vi "MoD Main-Optimize - HPLC PhotoRedox.vi"() -> ()   [LabVIEW 2015]
uses:
  <vilib>/silver_ctls/ArrayMatrixCluster/Real Matrix NI_Silver.ctl
  <vilib>/ni845x/ni845x.llb/ni845xControl.ctl
  <vilib>/MakerHub/LINX/Public/Peripherals/Analog/Analog Read 1 Chan.vi
  <vilib>/MakerHub/LINX/Public/Peripherals/Analog/Analog Read N Chans.vi
  <vilib>/MakerHub/LINX/Public/Peripherals/PWM/PWM Set Duty Cycle 1 Chan.vi
  <vilib>/MakerHub/LINX/Public/Peripherals/Digital/Digital Write 1 Chan.vi
  <vilib>/MakerHub/LINX/Private/Local IO/LinxAnalogRead.vi
  <vilib>/MakerHub/LINX/Public/Utilities/Check Channel.vi
  <vilib>/MakerHub/LINX/Public/Peripherals/Digital/Digital Write N Chans.vi
  <vilib>/MakerHub/LINX/Private/Local IO/LinxDigitalWrite.vi
  <vilib>/addons/control/pid/pid.llb/PID Control Input Filter (DBL).vi
  <vilib>/MakerHub/LINX/Private/Utilties/Generate Error.vi
  <vilib>/addons/control/pid/autopid.llb/PID Online Autotuning (Relay Feedback).vi
  <vilib>/Analysis/Matrix/Numeric/Conversions/Array To Matrix - RA2.vi
  <vilib>/MakerHub/LINX/Public/Peripherals/PWM/PWM Set Duty Cycle N Chans.vi
  <vilib>/ni845x/ni845x.llb/NI-845x Close Device Reference.vi
  <vilib>/addons/control/pid/NI_PID_autopid.lvlib
  <vilib>/addons/control/pid/NI_PID_pid.lvlib
  <vilib>/Analysis/Matrix/NI_Matrix.lvlib
  <vilib>/MakerHub/LINX/LMH-LINX.lvlib
  <instrlib>/Harvard Apparatus PHD Ultra Series/Harvard Apparatus PHD Ultra Series.lvlib
panel:
  out "running?":bool=TRUE
  out "new_reactor_volume":bool[](array[boolean])
  out "new_reactor_length":bool[](array[boolean])
  out "Phase_Sensor_voltage":dbl
  out "P_tot":dbl
  out "pause for ms":bool=TRUE
  out "stop_xl_write":bool=TRUE
  out "Num_exp_till_pause":i32
  out "Syringe_pump?":bool=TRUE
  out "System Error":bool=TRUE
  out "error out":errorcluster
  out "Pump setpoint(ul/min) 6":dbl format="%#_13g"
  out "Pump setpoint(ul/min) 5":dbl format="%#_13g"
  out "Pump setpoint(ul/min) 4":dbl format="%#_13g"
  out "Pump setpoint(ul/min) 3":dbl format="%#_13g"
  out "Pump setpoint(ul/min) 2":dbl format="%#_13g"
  out "Pump setpoint(ul/min) 1":dbl format="%#_13g"
  out "Volume (ul) 5":dbl format="%#_13g"
  out "Volume (ul) 4":dbl format="%#_13g"
  out "Volume (ul) 3":dbl format="%#_13g"
  out "Volume (ul) 2":dbl format="%#_13g"
  out "Volume (ul) 1":dbl format="%#_13g"
  in  "tau 5":dbl format="%#_13g"
  out "tau 4":dbl format="%#_13g"
  out "tau 3":dbl format="%#_13g"
  out "tau 2":dbl format="%#_13g"
  out "tau 1":dbl format="%#_13g"
  out "Reactor Length":dbl format="%#_13g"
  out "Flowrate Sensor 2":dbl format="%#_13g"
  out "Flowrate Sensor 1":dbl format="%#_13g"
  out "Pressure 2":dbl format="%#_13g"
  out "Pressure 1":dbl format="%#_13g"
  out "Temperature Control 5":bool=TRUE
  out "Temperature Control 4":bool=TRUE
  out "Temperature Control 3":bool=TRUE
  out "Temperature Control 2":bool=TRUE
  out "Temperature Control 1":bool=TRUE
  out "Temperature SP 5":dbl format="%#_g'C"
  out "Temperature SP 4":dbl format="%#_g'C"
  out "Temperature SP 3":dbl format="%#_g'C"
  out "Temperature SP 2":dbl format="%#_g'C"
  out "Temperature SP 1":dbl format="%#_g'C"
  in  "Bay Temperature 5":dbl
  in  "SSR Duration 5":dbl
  in  "SSR Duration 4":dbl
  in  "SSR Duration 3":dbl
  in  "SSR Duration 2":dbl
  in  "SSR Duration 1":dbl
  in  "Total Product Amount":dbl=1.0 format="%#_gml"
  out "Setup Error":bool=TRUE
  out "Error Message":string
  out "ID CTR":i32
  in  "Tab Control":T1(tab)
  out "Reagent pic 5":picture
  in  "reagent name 5":string
  out "Reagent Pic 4":picture
  in  "reagent name 4":string="Sodium cyanide"
  out "Reagent Pic 3":picture
  in  "reagent  name 3":string="50525-27-4"
  in  "Product name":string="55662-89-0"
  in  "reagent name 1":string="3340-78-1"
  out "Reagent Pic 1":picture
  in  "Vr5":dbl format="%#_guL"
  in  "Vr4":dbl format="%#_guL"
  in  "Vr3":dbl format="%#_guL"
  in  "Vr2":dbl format="%#_guL"
  in  "Vr1":dbl format="%#_guL"
  in  "System decide help Button":bool
  in  "Reaction Scheme Confirm":bool
  in  "Synthesis Route Array":string[][](array[string])=[["tetrahydroisoquinoline +IS(0.5M)", ".2", "PhB(OH)2", "", "", ""], ["BrCCl3", ".5", "-", "-", "-", "-"], ["Ru(bpy)3Cl2", "0.002", "-", "-", "-", "-"], ["NaCN", "4", "-", "-", "-", "-"], ["", "", "-", "-", "-", "-"], ["", "", "-", "-", "-", "-"]]
  in  "System decide help Button 2":bool
  out "Setup Confirm":bool=TRUE
  in  "BAY 1":u16(ring) items=["               Bypass", "         Heated Reactor", "    Small Heated Reator", "         Cooled Reactor", "      Packed Bed Reactor", "          Photo Reactor", "             Separator"]
  in  "BAY 5":u16(ring) items=["               Bypass", "         Heated Reactor", "    Small Heated Reactor", "         Cooled Reactor", "     Packed Bed Reactor", "         Photo Reactor", "             Separator"]
  in  "BAY 4":u16(ring) items=["                Bypass", "         Heated Reactor", "    Small Heated Reactor", "         Cooled Reactor", "     Packed Bed Reactor", "         Photo Reactor", "             Separator"]
  in  "BAY 3":u16(ring)=2 items=["               Bypass", "         Heated Reactor", "    Small Heated Reactor", "         Cooled Reactor", "     Packed Bed Reactor", "          Photo Reactor", "             Separator"]
  in  "BAY 2":u16(ring)=5 items=["               Bypass", "         Heated Reactor", "    Small Heated Reactor", "         Cooled Reactor", "      Packed Bed Reactor", "          Photo Reactor", "             Separator"]
  out "Reagent Pic 2":picture
  out "Product Pic":picture
  in  "reagent name 2":string="Bromotrichloromethane"
  in  "reagent name 6":string
  out "Reagent Pic 6":picture
  in  "System Parameters Help Button":bool
  out "Setup Confirm 2":bool
  in  "System Parameters Confirm Button":bool
  in  "Bay Parameters":T2={"Bay 1 "={"Pump 1 Flowrate"=0.0, "optimize_temp"=FALSE, "optimize_tau"=TRUE, "Run at set flowrate"=FALSE, "Pump 2 Flowrate"=0.0, "Temperature Params"=[40.0, 100.0, 100.0], "pump params 1"=[57.0, 122.0, 325.0], "pump params 2"=[57.0, 122.0, 325.0], "Temperature"=0.0, "Run at set temperature"=FALSE}, "Bay 2 "={"Pump 3 Flowrate"=0.0, "optimize_temp"=FALSE, "optimize_tau"=TRUE, "Run at set flowrate"=FALSE, "Temperature Params"=[40.0, 100.0, 100.0], "Resisdence time params"=[1.0, 5.0, 650.0], "pump_at_ratio"=FALSE, "pump_num_ratio"=4.0, "Temperature"=0.0, "Run at set temperature"=FALSE}, "Bay 3 "={"Pump 4 Flowrate"=100.0, "optimize_temp"=FALSE, "optimize_tau"=FALSE, "Run at set flowrate"=FALSE, "Temperature Params"=[40.0, 100.0, 100.0], "Resisdence time params"=[16.3, 65.9, 0.0], "pump_at_ratio"=TRUE, "pump_num_ratio"=0.05, "Temperature "=0.0, "Run at set temperature"=FALSE}, "Bay 4 "={"Pump 5 Flowrate"=40.0, "Run at set flowrate"=FALSE, "optimize_temp"=FALSE, "optimize_tau"=FALSE, "Resisdence time params"=[40.6, 406.0, 225.0], "Temperature Params"=[40.0, 100.0, 80.0], "pump_at_ratio"=FALSE, "pump_num_ratio"=1.0, "Temperature"=0.0, "Run at set temperature"=FALSE}, "Bay 5 "={"Pump 6 Flowrate"=0.0, "Run at set flowrate"=FALSE, "optimize_temp"=FALSE, "optimize_tau"=FALSE, "Resisdence time params"=[7.62, 114.27, 0.0], "Temperature Params"=[0.0, 0.0, 0.0], "pump_at_ratio"=FALSE, "pump_num_ratio"=0.5, "Temperature"=0.0, "Run at set temperature"=FALSE}, "Excel File Name"="C:\\Users\\HPLC\\Dropbox (MIT)\\MoD Files\\Data\\Photo08252017", "hplc File Name"="C:\\Chem32\\1\\Data\\MOD", "Matlab File"="C:\\Users\\HPLC\\Dropbox (MIT)\\MoD Files\\Data\\Photo08252017_1", "Syringe for Pump 2?"=TRUE, "Num_conditons_per_wait"=2.0, "Continue from previous optimization?"=FALSE, "Total Number of Experiments 2"=33.0, "Hplc Wait time(min)"=8.0, "increas_decrease_hplc_peak"=TRUE, "Internal Standard?"=TRUE, "ISTD start"=3.0, "ISTD end"=4.0, "hplc_start"=6.0, "hplc_end"=7.0, "throughput_yield"=FALSE} {"Hplc Wait time(min)" format="%#_13g"; "Bay 5"."Temperature Params" format="%#_g'C"; "Bay 4"."Temperature Params" format="%#_g'C"; "Bay 3"."Temperature Params" format="%#_g'C"; "Bay 2"."Temperature Params" format="%#_g'C"; "Bay 1"."Temperature Params" format="%#_g'C"}
  out "System Confirm Not Clicked":string
  out "best_exp_num":dbl=1.0
  out "temperature_best":dbl[](array[numeric])
  out "Flowrates(ul/min)_best":dbl[](array[numeric])
  out "System Status":u16(ring)=2 caption="Sy" items=["System  Error", "System Running", "System Standby"]
  out "Current Experiment":dbl=1.0
  out "Total Number of Experiments":dbl=33.0
  out "Phase Sensor Chart":T3(graph)
  out "HPLC Analysis":bool
  out "Equlibrating Temperature":bool
  out "Flushing System":bool
  out "Calculate condition":bool
  out "Temperature 5":dbl format="%#_g'C"
  out "Temperature 4":dbl format="%#_g'C"
  out "Temperature 3":dbl format="%#_g'C"
  out "Temperature 2":dbl format="%#_g'C"
  out "Temperature 1":dbl format="%#_g'C"
  out "Flowrate Chart":T4(graph)
  out "Teperature Chart":T3(graph)
  out "Pump Setpoints Chart":T3(graph)
  out "Pressure Chart":T3(graph)
  out "Optimization_loop_index":i32
  out "curr_wait_time":dbl
  out "total_flush_time":dbl
  out "Temp SS? 5":bool=TRUE
  out "Temp SS? 4":bool=TRUE
  out "Temp SS? 3":bool=TRUE
  out "Temp SS? 2":bool=TRUE
  out "Temp SS? 1":bool=TRUE
  out "System Flushed?":bool
  out "stop_button clicked":bool
  out "experiment history":T5
  in  "Number of System Flushes per condtion":dbl=1.5
  in  "calculate volume 3":bool=TRUE
  in  "calculate volume 2":bool=TRUE
  in  "calculate volume 1":bool=TRUE
  in  "calculate volume 4":bool
  in  "calculate volume 5":bool
  in  "Extra system dead volume":dbl format="%#_gul"
  in  "new reactor length? 1":bool
  in  "tube_length(in)":dbl[](array[numeric])=[188.0, 188.0, 10.0, 10.0, 10.0]
  out "Pause Before Analysis":bool
  out "Chiller COMM Port":bool
  out "Arduino COMM Port 2":bool
  out "Temperature Sensor COMM Port":bool
  out "Flow Rate":bool
  out "Pressure":bool
  out "Pump COMM Port":bool
  in  "COMM Port :: Milligat Pumps":refnum<visa-resource-name>="COM10"
  in  "Arduino COMM Port":refnum<visa-resource-name>="COM3"
  in  "Sample Valve COMM::Port":refnum<visa-resource-name>="COM4"
  in  "COMM Port:: Harvard Syringe Pump":refnum<visa-resource-name>="COM5"
  in  "tube_id(in)":enum16{".01", ".02", ".03", ".04"}[](array[ring])=[enum.".03", enum.".03", enum.".03", enum.".03", enum.".03"]
  out "Total System Resisdence Time(min)":dbl
  in  "Debug_run_button":bool
  in  "new reactor length? 2":bool
  in  "new reactor length? 3":bool
  in  "new reactor length? 4":bool
  in  "new reactor length? 5":bool
  in  "IR Sensor Device":T6="USB0::0x3923::0x7514::01B3FF21::RAW"
  out "Stop":bool=TRUE
  in  "Run_Stop_cluster":T7
  # "Molecules on Demand"
  # "Synthetic Route"
  # "5"
  # "6"
  # "4"
  # "Product"
  # "1"
  # "2"
  # "3"
  # "Reagent List"
  # "Concentration(M)"
  # "Molecule"
  # "1"
  # "1"
  # "2"
  # "2"
  # "3"
  # "3"
  # "4"
  # "4"
  # "5"
  # "6"
  # "5"
  # "6"
  # "Product"
  # "Reactor Volume:"
  # "Optimization Parameters"
  # "Pause after"
  # "Experiments"
  # "Optimize for"
  # "to"
  # "of HPLC Peak from"
  # "from"
  # "to"
  # "min"
  # "min"
  # "HPLC runtime"
  # "# Iterations"
  # "Reporting"
  # "Excel Output File Name"
  # "HPLC File Path"
  # "MATLAB File Path"
  # "Temperature"
  # "Flowrate(ul/min)"
  # "Lower Bound"
  # "Upper Bound"
  # "Optimize?"
  # "-or-"
  # "Run at"
  # "times incoming flow"
  # "Setpoint"
  # "Temperature"
  # "Flowrate(ul/min)"
  # "Lower Bound"
  # "Upper Bound"
  # "Optimize?"
  # "-or-"
  # "Run at"
  # "times incoming flow"
  # "Setpoint"
  # "Temperature"
  # "Flowrate(ul/min)"
  # "Lower Bound"
  # "Upper Bound"
  # "Optimize?"
  # "-or-"
  # "Run at"
  # "times incoming flow"
  # "Setpoint"
  # "Temperature"
  # "Flowrate 3 (ul/min)"
  # "Lower Bound"
  # "Upper Bound"
  # "Optimize?"
  # "-or-"
  # "Run at"
  # "times incoming flow"
  # "Setpoint"
  # "Temperature"
  # "Flowrate 1(ul/min)"
  # "Flowrate 2(ul/min)"
  # "Lower Bound"
  # "Upper Bound"
  # "Optimize?"
  # "Setpoint"
  # "Pressure (psi)"
  # "System Status"
  # "Temperature('C)"
  # "BAY"
  # "1"
  # "2"
  # "3"
  # "4"
  # "5"
  # "Pump Flowrate Setpoint(ul/min)"
  # "Flowrate (ul/min)"
  # "Phase Sensor"
  # "Current Experiment"
  # "Temperature('C)"
  # "Flowrate(ul/min)"
  # "Exp"
  # "Current Best Condition"
  # "Time to reach steady state:"
  # "Current Wait Time:"
  # "Experimental Steps"
  # "Calculated New Conditions"
  # "Steady State"
  # "Analyzed HPLC"
  # "Equilibrated Temperature"
  # "Tube Length (cm)"
  # "Bay"
  # "Tube ID (in)"
  # "Calculate Volume"
  # "Use new tube length"
  # "1."
  # "2."
  # "3."
  # "4."
  # "5."
  # "Reactor Lengths\n*Heated Reactor - 188cm * Small Reactor - 99cm * Bypass - 10cm * Separator - *"
  # "All Experimental Data"
  # "P1"
  # "P2"
  # "P3"
  # "P4"
  # "P5"
  # "P6"
  # "T1"
  # "T2"
  # "T3"
  # "T4"
  # "T5"
  # "Obj_fun"
  # "HPLC_Data"
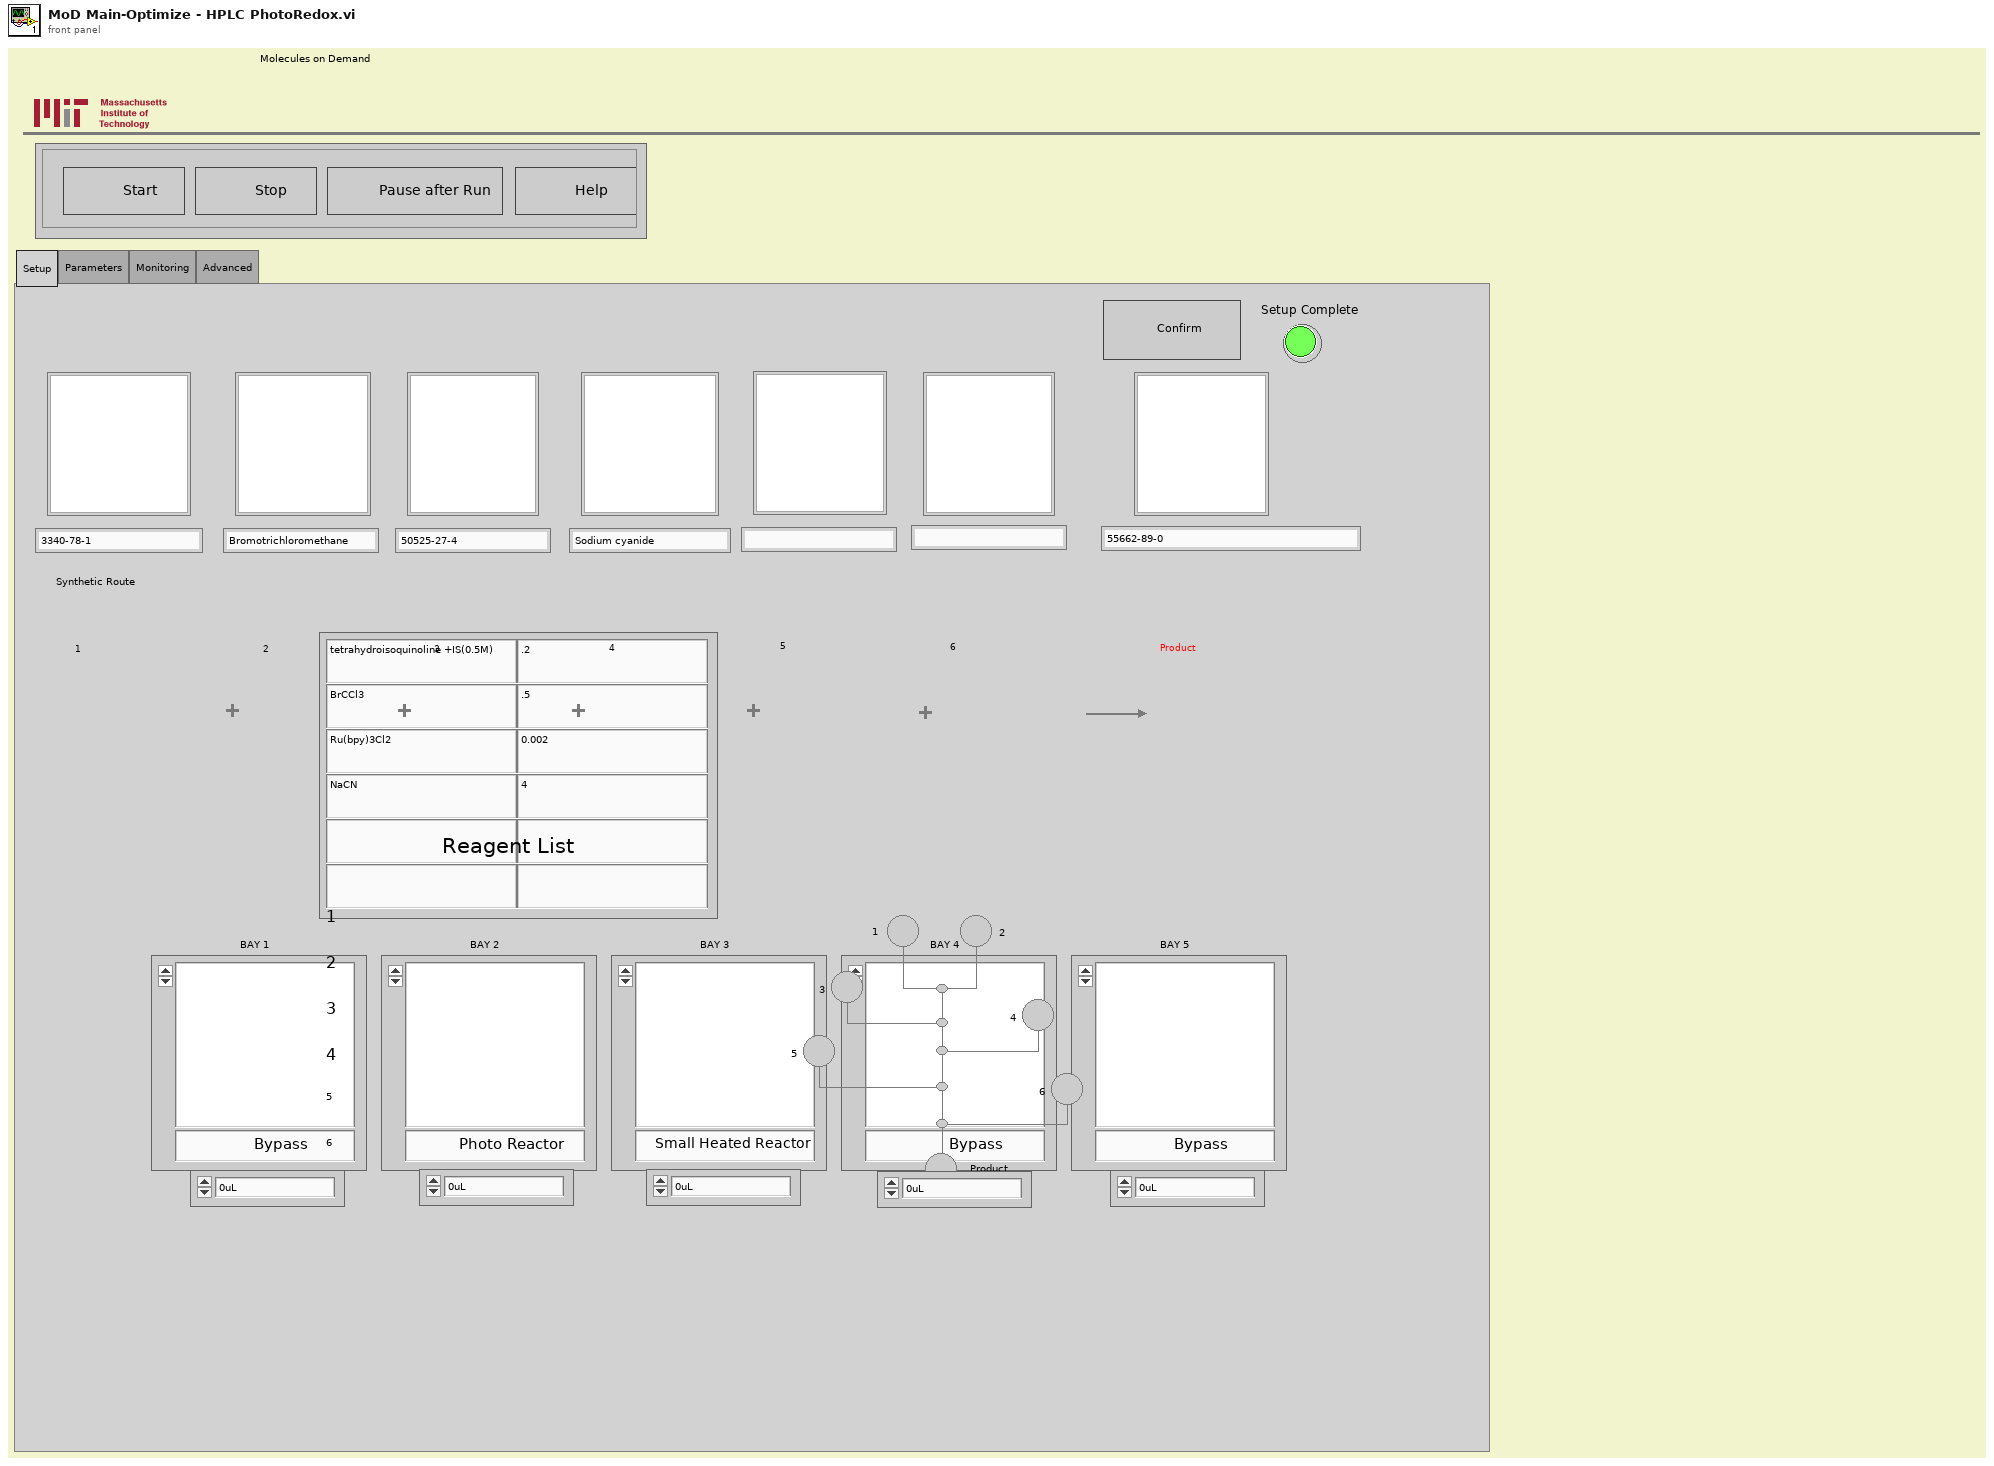
[diagram p1: front panel]
types:
  T1 = enum32{"Setup", "Parameters", "Monitoring", "Advanced"}
  T2 = cluster{"Bay 1 ":cluster{"Pump 1 Flowrate":dbl, "optimize_temp":bool, "optimize_tau":bool, "Run at set flowrate":bool, "Pump 2 Flowrate":dbl, "Temperature Params":dbl[], "pump params 1":dbl[], "pump params 2":dbl[], "Temperature":dbl, "Run at set temperature":bool}, "Bay 2 ":cluster{"Pump 3 Flowrate":dbl, "optimize_temp":bool, "optimize_tau":bool, "Run at set flowrate":bool, "Temperature Params":dbl[], "Resisdence time params":dbl[], "pump_at_ratio":bool, "pump_num_ratio":dbl, "Temperature":dbl, "Run at set temperature":bool}, "Bay 3 ":cluster{"Pump 4 Flowrate":dbl, "optimize_temp":bool, "optimize_tau":bool, "Run at set flowrate":bool, "Temperature Params":dbl[], "Resisdence time params":dbl[], "pump_at_ratio":bool, "pump_num_ratio":dbl, "Temperature ":dbl, "Run at set temperature":bool}, "Bay 4 ":cluster{"Pump 5 Flowrate":dbl, "Run at set flowrate":bool, "optimize_temp":bool, "optimize_tau":bool, "Resisdence time params":dbl[], "Temperature Params":dbl[], "pump_at_ratio":bool, "pump_num_ratio":dbl, "Temperature":dbl, "Run at set temperature":bool}, "Bay 5 ":cluster{"Pump 6 Flowrate":dbl, "Run at set flowrate":bool, "optimize_temp":bool, "optimize_tau":bool, "Resisdence time params":dbl[], "Temperature Params":dbl[], "pump_at_ratio":bool, "pump_num_ratio":dbl, "Temperature":dbl, "Run at set temperature":bool}, "Excel File Name":string, "hplc File Name":string, "Matlab File":string, "Syringe for Pump 2?":bool, "Num_conditons_per_wait":dbl, "Continue from previous optimization?":bool, "Total Number of Experiments 2":dbl, "Hplc Wait time(min)":dbl, "increas_decrease_hplc_peak":bool, "Internal Standard?":bool, "ISTD start":dbl, "ISTD end":dbl, "hplc_start":dbl, "hplc_end":dbl, "throughput_yield":bool}
  T3 = cluster{"[0]":dbl, "[1]":dbl, "[2]":dbl, "[3]":dbl, "[4]":dbl, "[5]":dbl, "[6]":dbl, "[7]":dbl, "[8]":dbl}
  T4 = cluster{"[0]":i32, "[1]":i32, "[2]":i32, "[3]":i32, "[4]":i32, "[5]":i32, "[6]":i32, "[7]":i32, "[8]":i32}
  T5 = typedef "Real Matrix NI_Silver.ctl" = dbl[][]
  T6 = typedef "ni845xControl.ctl" = refnum<k21>
  T7 = cluster{"Stop":bool, "Run":bool, "Stop Run Button":bool, "Help Button":bool}
  T8 = cluster{"Proportional gain Kc":dbl, "Integral time Ti (sec)":dbl, "Derivative time Ti (sec)":dbl}
  T9 = cluster{"type of controller":enum16{"P", "PI", "PID"}, "relay cycles":i32, "relay amplitude":dbl, "control specifications":enum16{"Fast", "Normal", "Slow"}, "PV noise level":dbl}
  T10 = typedef "LMH-LINX.lvlib/LINX Ref.ctl" = cluster{"IO":T11, "Interface":T12, "LINX Device Config":T13}
  T11 = typedef "LMH-LINX.lvlib/Platform.ctl" = enum16{"Remote", "Local"}
  T12 = typedef "LMH-LINX.lvlib/Interface.ctl" = enum16{"Serial", "TCP"}
  T13 = typedef "LMH-LINX.lvlib/Device.lvlib/LINX Device Config.ctl" = cluster{"Interface":T12, "COM Port":refnum<visa-resource-name>, "TCP Configuration":T14, "Device Family":u8, "Device ID":u8, "Device Name":string, "TCP Ref":refnum<k5>, "Channels":T15}
  T14 = typedef "LMH-LINX.lvlib/Device.lvlib/TCP Config.ctl" = cluster{"IP Address":string, "Port":u16}
  T15 = typedef "LMH-LINX.lvlib/Channels.ctl" = cluster{"DI":u8[], "DO":u8[], "AI":u8[], "AO":u8[], "PWM":u8[], "QE":u8[], "UART":u8[], "I2C 2":u8[], "SPI":u8[], "CAN":u8[], "Servo":u8[], "AI Ref (V)":dbl, "AI Resolution (Bits)":u8, "AO Ref (V)":dbl, "AO Resolution (Bits)":u8}
  T16 = typedef "imagedata.ctl" = cluster{"image type":i32, "image depth":i32, "image":u8[], "mask":u8[], "colors":u32[], "Rectangle":cluster{"left":i16, "top":i16, "right":i16, "bottom":i16}}
  T17 = cluster{"proportional gain (Kc)":dbl, "integral time (Ti, min)":dbl, "derivative time (Td, min)":dbl}
  T18 = typedef "NI_Matrix.lvlib/RealMatrix.ctl" = dbl[][]
  T19 = enum16{"Left Button", "Center Button", "Right Button", "Window Close"}
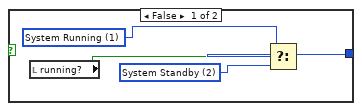
[diagram p4: hidden frame]
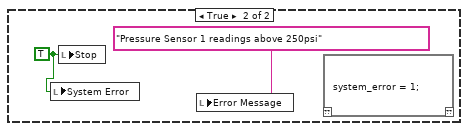
[diagram p6: hidden frame]
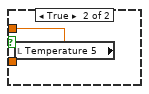
[diagram p7: hidden frame]
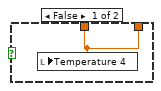
[diagram p8: hidden frame]
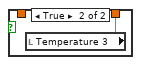
[diagram p9: hidden frame]
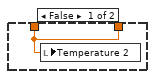
[diagram p10: hidden frame]
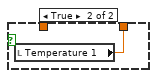
[diagram p11: hidden frame]
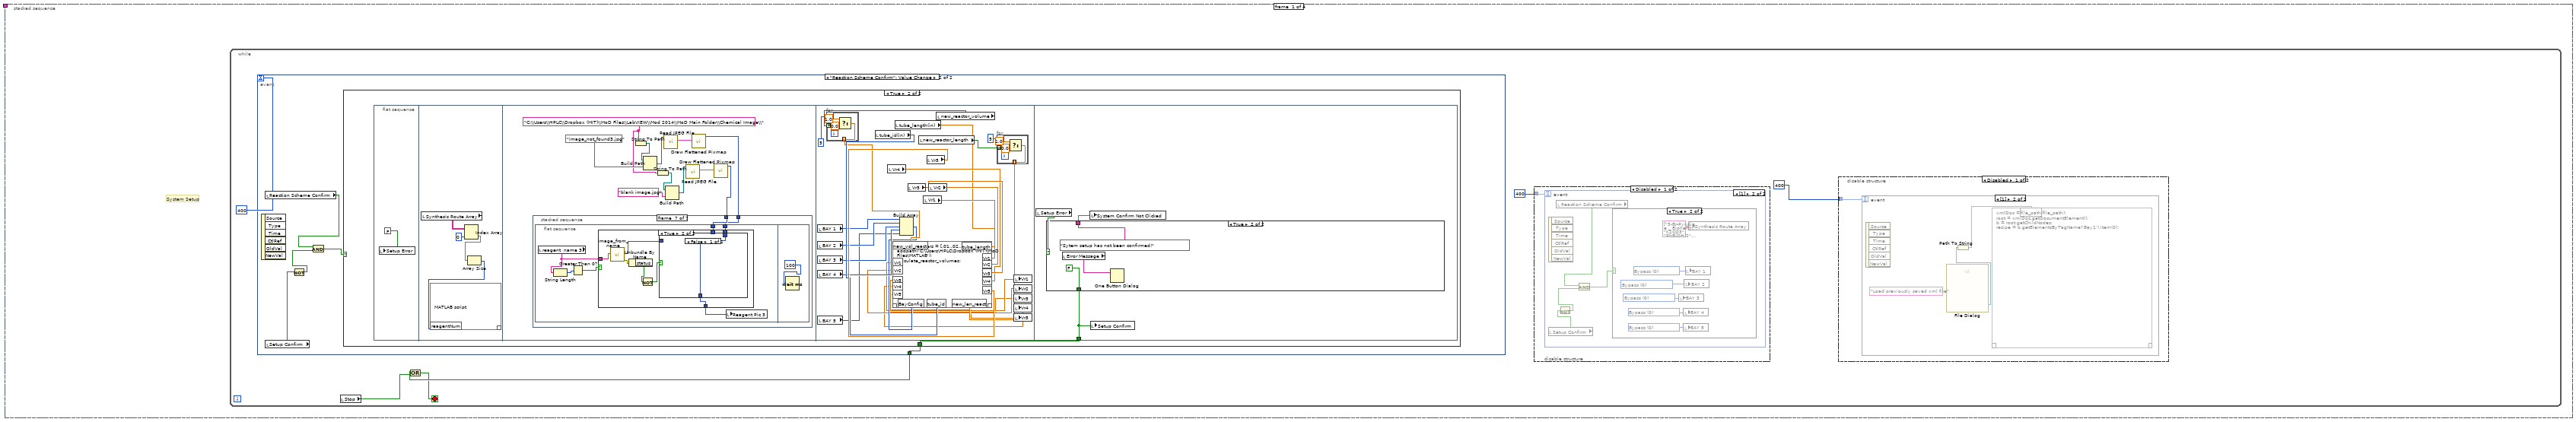
[diagram p12: hidden frame]
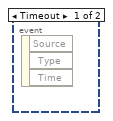
[diagram p13: hidden frame]
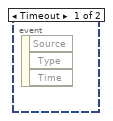
[diagram p15: hidden frame]
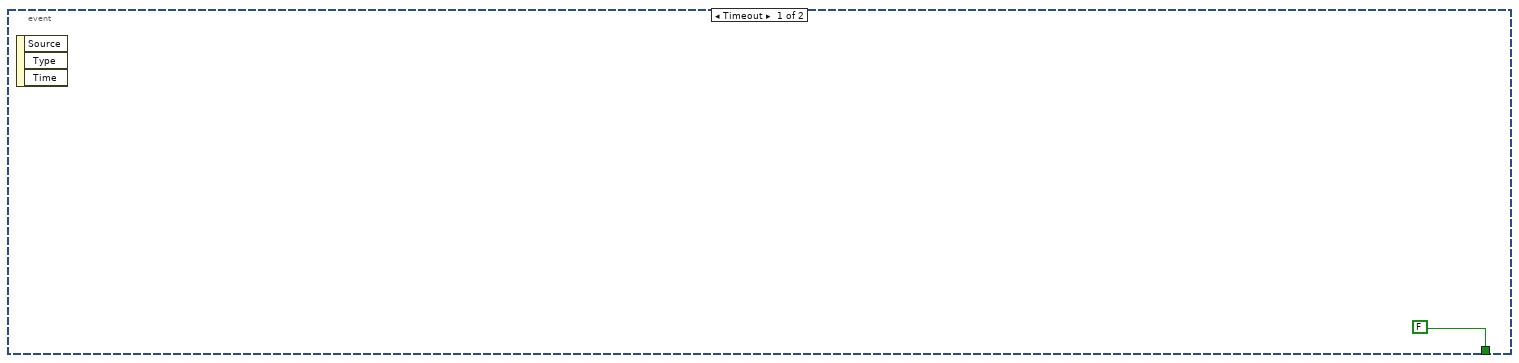
[diagram p18: hidden frame]
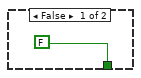
[diagram p19: hidden frame]
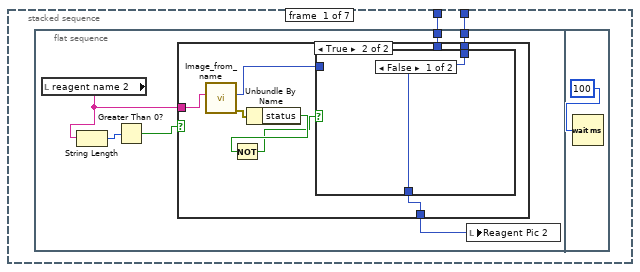
[diagram p20: hidden frame]
diagram:
  # "Assume User always uses the first bay first"
  n1 = flat-sequence {
    tunnel: ["COMM Port :: Milligat Pumps"] -> w9
    tunnel: ["Arduino COMM Port"] -> w8
    tunnel: [w11] -> w5
    tunnel: ["Bay Parameters"] -> w4
    tunnel: [w60] -> w10
    tunnel: w9 -> [w60]
    tunnel: w8 -> [w48]
    tunnel: [w54] -> w7
    tunnel: [w52] -> w6
    tunnel: w5 -> [w52]
    tunnel: w4 -> [w50]
    tunnel: [w47] -> w3
    tunnel: w10 -> [w66]
    tunnel: w7 -> [w65]
    tunnel: w6 -> [w63]
    tunnel: w3 -> [w61]
    tunnel: [w61] -> w1
    tunnel: [w1380] -> w2
    tunnel: w1 -> [w1380]
    tunnel: w2 -> [w1381]
    frame #0 {
      w36 = FALSE ("Equlibrating Temperature")
      n2 = script code="TempArr1=[23 23 23 23 23 23 23 23 23 23]';\nTempArr2=[23 23 23 23 23 23 23 23 23 23]';\nTempArr3=[23 23 23 23 23 23 23 23 23 23]';\nTempArr4=[23 23 23 23 23 23 23 23 23 23]';\nTempArr5=[23 23 23 23 23 23 23 23 23 23]';\nTempArrLED=[23 23 23 23 23 23 23 23 23 23]';\ntemp_error1 =0;\ntemp_error2 =0;\ntemp_error3 =0;\ntemp_error4 =0;\ntemp_error5 =0;\ntemp_check1 = 0;\ntemp_check2 = 0;\ntemp_check3 = 0;\ntemp_check4 = 0;\ntemp_check5 = 0;\nT1=23;\nT2=23;\nT3=23;\nT4=23;\nT5=23;"() -> ()  [unwired: 1 in, 1 out]
      n3 = Build Array("calculate volume 1", "calculate volume 2", "calculate volume 3", "calculate volume 4", "calculate volume 5") -> (→"new_reactor_volume":bool[])
      n4 = Build Array("new reactor length? 1", "new reactor length? 2", "new reactor length? 3", "new reactor length? 4", "new reactor length? 5") -> (→"new_reactor_length":bool[])
      n5 = call <vilib>:"Initialize.vi"("VISA resource name"="COMM Port:: Harvard Syringe Pump") -> ("VISA resource name out"=w11:refnum<visa-resource-name>)  [unwired: 9 in, 1 out]
      "Stop" <- FALSE ("Stop")
      "ID CTR" <- 0
      "Setup Confirm" <- FALSE ("Setup Confirm")
      "Error Message" <- "System shutdown sucessfully. No errors to report." ("Error Message")
      "Setup Error" <- FALSE ("Setup Error")
      "Reactor Length" <- 10.5
      "System Error" <- FALSE ("System Error")
      "Num_exp_till_pause" <- 0 ("Num_exp_till_pause")
      "Equlibrating Temperature" <- w36
      "Calculate condition" <- w36
      "Flushing System" <- w36
      "HPLC Analysis" <- w36
      "stop_xl_write" <- FALSE ("stop_xl_write")
      "Pump setpoint(ul/min) 1" <- 0.0 ("Pump setpoint(ul/min) 1")
      "Pump setpoint(ul/min) 2" <- 0.0 ("Pump setpoint(ul/min) 2")
      "Pump setpoint(ul/min) 4" <- 0.0 ("Pump setpoint(ul/min) 4")
      "Pump setpoint(ul/min) 6" <- 0.0 ("Pump setpoint(ul/min) 6")
      "Pump setpoint(ul/min) 3" <- 0.0 ("Pump setpoint(ul/min) 3")
      "Pump setpoint(ul/min) 5" <- 0.0 ("Pump setpoint(ul/min) 5")
      "pause for ms" <- FALSE ("pause for ms")
      "Setup Confirm 2" <- FALSE ("Setup Confirm 2")
      "running?" <- FALSE ("running?")
    }
    frame #1 {
      w49 = FALSE
      w59 = 23
      (unwired) path "C:/Users/User1/Documents/Lab/MoD/Images"
      n6 = disable-structure shown="Disabled" {
        frame Disabled {
          n7 = local read "BAY 2"() -> ()  [unwired: 1 out]
          n8 = local read "BAY 3"() -> ()  [unwired: 1 out]
          n9 = local read "BAY 4"() -> ()  [unwired: 1 out]
          n10 = local read "BAY 5"() -> ()  [unwired: 1 out]
          n11 = local read "BAY 1"() -> ()  [unwired: 1 out]
        }
        frame Enabled {
        }
      }
      n12 = local write "Debug_run_button"(TRUE) -> ()
      n13 = call <vilib>:"Initialize.vi"("Serial Port"=w48) -> ("LINX Resource"=w47:T10)  [unwired: 8 in, 2 out]
      n14 = local write "System Parameters Confirm Button"(w49) -> ()
      n15 = local write "Setup Confirm 2"(w49) -> ()
      n16 = Unbundle By Name(w50) -> ("Syringe for Pump 2?"=→"Syringe_pump?":bool)
      n17 = local write "Temperature 1"(w59) -> ()
      n18 = local write "Temperature 2"(w59) -> ()
      n19 = local write "Temperature 3"(w59) -> ()
      n20 = local write "Temperature 4"(w59) -> ()
      n21 = local write "Temperature 5"(w59) -> ()
      n22 = local write "Temperature SP 1"(w59) -> ()
      n23 = local write "Temperature SP 2"(w59) -> ()
      n24 = local write "Temperature SP 3"(w59) -> ()
      n25 = local write "Temperature SP 4"(w59) -> ()
      n26 = local write "Temperature SP 5"(w59) -> ()
      n27 = Current VI's Path() -> (path=w58:path)
      n28 = Strip Path(path=w58) -> (stripped path=w56:path)  [unwired: 1 out]
      n29 = Strip Path(path=w56) -> (stripped path=w55:path)  [unwired: 1 out]
      n30 = Build Path(base path=w55, name or relative path="MATLAB") -> (appended path=w54:path)
    }
    frame #2 {
      # "Main Help Dialog Popup"
      n31 = while {
        stop <- w1374 stop-if-true
        n32 = event shown="[6] \"Run_Stop_cluster.Run\": Value Change" {
          selector: _ -> [_ _ _ _ _ _ _]
          dyn-events: _ -> [_ _ _ _ _ _ _]
          timeout: 100 -> [_ _ _ _ _ _ _]
          event Timeout {
            n33 = event-data() -> ()  [unwired: 1 in, 3 out]
          }
          event "Run_Stop_cluster.Help Button": Value Change {
            n34 = local read "Run_Stop_cluster"() -> (w1377:T7)
            n35 = event-data() -> ()  [unwired: 1 in, 4 out]
            n36 = Unbundle By Name(w1377) -> ("Help Button"=w1376:bool)
            n37 = case shown="True" w1376 {
              frame False {
              }
              frame True {
                n38 = call "help.vi"() -> ()  [unwired: 11 in]
              }
            }
          }
          event "System decide help Button": Value Change {
            n39 = event-data() -> ()  [unwired: 1 in, 5 out]
            n40 = call "help_synthesis_man-auto_instructions.vi"() -> ()  [unwired: 12 in]
          }
          event "System Parameters Help Button": Value Change {
            n41 = event-data() -> ()  [unwired: 1 in, 5 out]
            n42 = call "help_parameters_setup.vi"() -> ()  [unwired: 12 in]
          }
          event "System decide help Button 2": Value Change {
            n43 = event-data() -> ()  [unwired: 1 in, 5 out]
            n44 = call "help_synthesis_route_instructions.vi"() -> ()  [unwired: 12 in]
          }
          event "Run_Stop_cluster.Stop": Value Change {
            n45 = event-data() -> ()  [unwired: 1 in, 5 out]
            n46 = local write "Stop"(TRUE) -> ()
          }
          event "Run_Stop_cluster.Run": Value Change {
            n47 = event-data() -> ()  [unwired: 1 in, 5 out]
            n48 = local write "running?"(TRUE) -> ()
          }
        }
        n49 = local read "Stop"() -> (w1374:bool)
      }
      n50 = stacked-sequence {
        tunnel: w66 -> [_ _ _ _]
        tunnel: w65 -> [_ w432 _ _]
        tunnel: w63 -> [_ _ _ w599]
        tunnel: w61 -> [_ _ _ w597]
        frame #0 {
          # "System Setup"
          n51 = while {
            stop <- w207 stop-if-true
            n52 = event shown="[1] \"Reaction Scheme Confirm\": Value Change" {
              selector: _ -> [_ _]
              dyn-events: _ -> [_ _]
              timeout: 400 -> [_ _]
              tunnel: [FALSE w227] -> w209
              event Timeout {
                n53 = event-data() -> ()  [unwired: 1 in, 3 out]
              }
              event "Reaction Scheme Confirm": Value Change {
                n54 = event-data() -> ()  [unwired: 1 in, 6 out]
                n55 = local read "Reaction Scheme Confirm"() -> (w231:bool)
                n56 = local read "Setup Confirm"() -> (w229:bool)
                n57 = Not(x=w229) -> (.not. x?=w228:bool)
                n58 = And(x=w231, y=w228) -> (x .and. y?=w230:bool)
                n59 = case shown="True" w230 {
                  tunnel: [FALSE w233] -> w227
                  frame False {
                  }
                  frame True {
                    n60 = flat-sequence {
                      tunnel: [w422] -> w233
                      frame #0 {
                        n61 = local write "Setup Error"(FALSE) -> ()
                      }
                      frame #1 {
                        n62 = local read "Synthesis Route Array"() -> (w237:string[][])
                        n63 = Index Array(array=w237, index (col)=0 ("disabled index (col)")) -> (element=w235:string[])  [unwired: 1 in]
                        n64 = Array Size(array=w235) -> (size(s)=w238:i32)
                        n65 = script code="MATLAB script"("reagentNum"=w238) -> ()  [unwired: 1 in, 1 out]
                      }
                      frame #2 {
                        w241 = "C:\\Users\\HPLC\\Dropbox (MIT)\\MoD Files\\LabVIEW\\Mod 2014\\MoD Main Folder\\Chemical Image\\" ("string")
                        n66 = String To Path(string=w241) -> (path=w247:path)
                        n67 = Build Path(base path=w247, name or relative path="image_not_found3.jpg") -> (appended path=w246:path)
                        n68 = String To Path(string=w241) -> (path=w244:path)
                        n69 = call <vilib>:"Read JPEG File.vi"("path to JPEG file"=w246) -> ("image data"=w249:T16)  [unwired: 1 in, 9 out]
                        n70 = Build Path(base path=w244, name or relative path="blank image.jpg") -> (appended path=w242:path)
                        n71 = call <vilib>:"Read JPEG File.vi"("path to JPEG file"=w242) -> ("image data"=w245:T16)  [unwired: 1 in, 9 out]
                        n72 = call <vilib>:"Draw Flattened Pixmap.vi"("image data"=w249) -> ("new picture"=w240:picture)  [unwired: 3 in, 5 out]
                        n73 = call <vilib>:"Draw Flattened Pixmap.vi"("image data"=w245) -> ("new picture"=w239:picture)  [unwired: 3 in, 5 out]
                        n74 = stacked-sequence {
                          tunnel: w240 -> [w251 w271 w291 w311 w331 w350 w370]
                          tunnel: w239 -> [w250 w270 w290 w310 w330 w351 w371]
                          frame #0 {
                            n75 = flat-sequence {
                              tunnel: w251 -> [w257]
                              tunnel: w250 -> [w255]
                              frame #0 {
                                n76 = local read "reagent name 2"() -> (w253:string)
                                n77 = String Length(string=w253) -> (length=w256:i32)
                                n78 = Greater Than 0?(x=w256) -> (x > 0?=w254:bool)
                                n79 = case shown="True" w254 {
                                tunnel: w257 -> [_ w263]
                                tunnel: w255 -> [w258 _]
                                tunnel: [w258 w262] -> w252
                                tunnel: w253 -> [_ w261]
                                frame False {
                                }
                                frame True {
                                n80 = call "Image_from_name.vi"("Chemical Name"=w261) -> ("error out"=w264:errorcluster, "Downloaded Picture"=w265:picture)  [unwired: 8 in, 1 out]
                                n81 = Unbundle By Name(w264) -> ("status"=w260:bool)
                                n82 = Not(x=w260) -> (.not. x?=w259:bool)
                                n83 = case shown="False" w259 {
                                tunnel: w265 -> [_ w268]
                                tunnel: [w266 w267] -> w262
                                tunnel: w263 -> [w266 _]
                                frame False {
                                }
                                frame True {
                                n84 = call <vilib>:"Draw Flattened Pixmap.vi"("picture"=w268) -> ("new picture"=w267:picture)  [unwired: 8 in]
                                }
                                }
                                }
                                }
                                n85 = local write "Reagent Pic 2"(w252) -> ()
                              }
                              frame #1 {
                                n86 = Wait (ms)(milliseconds to wait=100) -> ()  [unwired: 1 out]
                              }
                            }
                          }
                          frame #1 {
                            n87 = flat-sequence {
                              tunnel: w271 -> [w277]
                              tunnel: w270 -> [w275]
                              frame #0 {
                                n88 = local read "reagent name 1"() -> (w272:string)
                                n89 = String Length(string=w272) -> (length=w276:i32)
                                n90 = Greater Than 0?(x=w276) -> (x > 0?=w274:bool)
                                n91 = case shown="True" w274 {
                                tunnel: w277 -> [_ w283]
                                tunnel: w275 -> [w278 _]
                                tunnel: [w278 w282] -> w273
                                tunnel: w272 -> [_ w281]
                                frame False {
                                }
                                frame True {
                                n92 = call "Image_from_name.vi"("Chemical Name"=w281) -> ("error out"=w284:errorcluster, "Downloaded Picture"=w285:picture)  [unwired: 8 in, 1 out]
                                n93 = Unbundle By Name(w284) -> ("status"=w280:bool)
                                n94 = Not(x=w280) -> (.not. x?=w279:bool)
                                n95 = case shown="True" w279 {
                                tunnel: w285 -> [_ w288]
                                tunnel: [w286 w287] -> w282
                                tunnel: w283 -> [w286 _]
                                frame False {
                                }
                                frame True {
                                n96 = call <vilib>:"Draw Flattened Pixmap.vi"("picture"=w288) -> ("new picture"=w287:picture)  [unwired: 8 in]
                                }
                                }
                                }
                                }
                                n97 = local write "Reagent Pic 1"(w273) -> ()
                              }
                              frame #1 {
                                n98 = Wait (ms)(milliseconds to wait=100) -> ()  [unwired: 1 out]
                              }
                            }
                          }
                          frame #2 {
                            n99 = flat-sequence {
                              tunnel: w291 -> [w297]
                              tunnel: w290 -> [w295]
                              frame #0 {
                                n100 = local read "Product name"() -> (w292:string)
                                n101 = String Length(string=w292) -> (length=w296:i32)
                                n102 = Greater Than 0?(x=w296) -> (x > 0?=w294:bool)
                                n103 = case shown="True" w294 {
                                tunnel: w297 -> [_ w303]
                                tunnel: w295 -> [w298 _]
                                tunnel: [w298 w302] -> w293
                                tunnel: w292 -> [_ w301]
                                frame False {
                                }
                                frame True {
                                n104 = call "Image_from_name.vi"("Chemical Name"=w301) -> ("error out"=w304:errorcluster, "Downloaded Picture"=w305:picture)  [unwired: 8 in, 1 out]
                                n105 = Unbundle By Name(w304) -> ("status"=w299:bool)
                                n106 = Not(x=w299) -> (.not. x?=w300:bool)
                                n107 = case shown="False" w300 {
                                tunnel: w305 -> [_ w308]
                                tunnel: [w306 w307] -> w302
                                tunnel: w303 -> [w306 _]
                                frame False {
                                }
                                frame True {
                                n108 = call <vilib>:"Draw Flattened Pixmap.vi"("picture"=w308) -> ("new picture"=w307:picture)  [unwired: 8 in]
                                }
                                }
                                }
                                }
                                n109 = local write "Product Pic"(w293) -> ()
                              }
                              frame #1 {
                                n110 = Wait (ms)(milliseconds to wait=100) -> ()  [unwired: 1 out]
                              }
                            }
                          }
                          frame #3 {
                            n111 = flat-sequence {
                              tunnel: w311 -> [w317]
                              tunnel: w310 -> [w315]
                              frame #0 {
                                n112 = local read "reagent name 6"() -> (w312:string)
                                n113 = String Length(string=w312) -> (length=w316:i32)
                                n114 = Greater Than 0?(x=w316) -> (x > 0?=w314:bool)
                                n115 = case shown="True" w314 {
                                tunnel: w317 -> [_ w323]
                                tunnel: w315 -> [w318 _]
                                tunnel: [w318 w322] -> w313
                                tunnel: w312 -> [_ w321]
                                frame False {
                                }
                                frame True {
                                n116 = call "Image_from_name.vi"("Chemical Name"=w321) -> ("error out"=w324:errorcluster, "Downloaded Picture"=w325:picture)  [unwired: 8 in, 1 out]
                                n117 = Unbundle By Name(w324) -> ("status"=w319:bool)
                                n118 = Not(x=w319) -> (.not. x?=w320:bool)
                                n119 = case shown="False" w320 {
                                tunnel: w325 -> [_ w328]
                                tunnel: [w326 w327] -> w322
                                tunnel: w323 -> [w326 _]
                                frame False {
                                }
                                frame True {
                                n120 = call <vilib>:"Draw Flattened Pixmap.vi"("picture"=w328) -> ("new picture"=w327:picture)  [unwired: 8 in]
                                }
                                }
                                }
                                }
                                n121 = local write "Reagent Pic 6"(w313) -> ()
                              }
                              frame #1 {
                                n122 = Wait (ms)(milliseconds to wait=100) -> ()  [unwired: 1 out]
                              }
                            }
                          }
                          frame #4 {
                            n123 = flat-sequence {
                              tunnel: w331 -> [w337]
                              tunnel: w330 -> [w335]
                              frame #0 {
                                n124 = local read "reagent name 5"() -> (w332:string)
                                n125 = String Length(string=w332) -> (length=w336:i32)
                                n126 = Greater Than 0?(x=w336) -> (x > 0?=w334:bool)
                                n127 = case shown="True" w334 {
                                tunnel: w337 -> [_ w343]
                                tunnel: w335 -> [w338 _]
                                tunnel: [w338 w342] -> w333
                                tunnel: w332 -> [_ w341]
                                frame False {
                                }
                                frame True {
                                n128 = call "Image_from_name.vi"("Chemical Name"=w341) -> ("error out"=w344:errorcluster, "Downloaded Picture"=w345:picture)  [unwired: 8 in, 1 out]
                                n129 = Unbundle By Name(w344) -> ("status"=w339:bool)
                                n130 = Not(x=w339) -> (.not. x?=w340:bool)
                                n131 = case shown="False" w340 {
                                tunnel: w345 -> [_ w348]
                                tunnel: [w346 w347] -> w342
                                tunnel: w343 -> [w346 _]
                                frame False {
                                }
                                frame True {
                                n132 = call <vilib>:"Draw Flattened Pixmap.vi"("picture"=w348) -> ("new picture"=w347:picture)  [unwired: 8 in]
                                }
                                }
                                }
                                }
                                n133 = local write "Reagent pic 5"(w333) -> ()
                              }
                              frame #1 {
                                n134 = Wait (ms)(milliseconds to wait=100) -> ()  [unwired: 1 out]
                              }
                            }
                          }
                          frame #5 {
                            n135 = flat-sequence {
                              tunnel: w351 -> [w355]
                              tunnel: w350 -> [w354]
                              frame #0 {
                                n136 = local read "reagent name 4"() -> (w352:string)
                                n137 = String Length(string=w352) -> (length=w357:i32)
                                n138 = Greater Than 0?(x=w357) -> (x > 0?=w356:bool)
                                n139 = case shown="True" w356 {
                                tunnel: w354 -> [_ w363]
                                tunnel: w355 -> [w358 _]
                                tunnel: [w358 w362] -> w353
                                tunnel: w352 -> [_ w361]
                                frame False {
                                }
                                frame True {
                                n140 = call "Image_from_name.vi"("Chemical Name"=w361) -> ("error out"=w364:errorcluster, "Downloaded Picture"=w365:picture)  [unwired: 8 in, 1 out]
                                n141 = Unbundle By Name(w364) -> ("status"=w359:bool)
                                n142 = Not(x=w359) -> (.not. x?=w360:bool)
                                n143 = case shown="False" w360 {
                                tunnel: w365 -> [_ w368]
                                tunnel: [w366 w367] -> w362
                                tunnel: w363 -> [w366 _]
                                frame False {
                                }
                                frame True {
                                n144 = call <vilib>:"Draw Flattened Pixmap.vi"("picture"=w368) -> ("new picture"=w367:picture)  [unwired: 8 in]
                                }
                                }
                                }
                                }
                                n145 = local write "Reagent Pic 4"(w353) -> ()
                              }
                              frame #1 {
                                n146 = Wait (ms)(milliseconds to wait=100) -> ()  [unwired: 1 out]
                              }
                            }
                          }
                          frame #6 {
                            n147 = flat-sequence {
                              tunnel: w371 -> [w375]
                              tunnel: w370 -> [w374]
                              frame #0 {
                                n148 = local read "reagent  name 3"() -> (w372:string)
                                n149 = String Length(string=w372) -> (length=w377:i32)
                                n150 = Greater Than 0?(x=w377) -> (x > 0?=w376:bool)
                                n151 = case shown="True" w376 {
                                tunnel: w374 -> [_ w383]
                                tunnel: w375 -> [w378 _]
                                tunnel: [w378 w382] -> w373
                                tunnel: w372 -> [_ w381]
                                frame False {
                                }
                                frame True {
                                n152 = call "Image_from_name.vi"("Chemical Name"=w381) -> ("error out"=w384:errorcluster, "Downloaded Picture"=w385:picture)  [unwired: 8 in, 1 out]
                                n153 = Unbundle By Name(w384) -> ("status"=w379:bool)
                                n154 = Not(x=w379) -> (.not. x?=w380:bool)
                                n155 = case shown="False" w380 {
                                tunnel: w385 -> [_ w388]
                                tunnel: [w386 w387] -> w382
                                tunnel: w383 -> [w386 _]
                                frame False {
                                }
                                frame True {
                                n156 = call <vilib>:"Draw Flattened Pixmap.vi"("picture"=w388) -> ("new picture"=w387:picture)  [unwired: 8 in]
                                }
                                }
                                }
                                }
                                n157 = local write "Reagent Pic 3"(w373) -> ()
                              }
                              frame #1 {
                                n158 = Wait (ms)(milliseconds to wait=100) -> ()  [unwired: 1 out]
                              }
                            }
                          }
                        }
                      }
                      frame #3 {
                        n159 = local read "BAY 1"() -> (w400:u16)
                        n160 = local read "BAY 2"() -> (w399:u16)
                        n161 = local read "BAY 3"() -> (w398:u16)
                        n162 = local read "BAY 4"() -> (w397:u16)
                        n163 = local read "BAY 5"() -> (w396:u16)
                        n164 = local read "tube_id(in)"() -> (w407:enum16{".01", ".02", ".03", ".04"}[])
                        n165 = local read "Vr4"() -> (w410:dbl)
                        n166 = local read "tube_length(in)"() -> (w408:dbl[])
                        n167 = Build Array(w400, w399, w398, w397, w396) -> (w395:u16[])
                        n168 = local read "Vr3"() -> (w411:dbl)
                        n169 = local read "new_reactor_length"() -> (w405:bool[])
                        n170 = local read "Vr1"() -> (w413:dbl)
                        n171 = local read "Vr5"() -> (w409:dbl)
                        n172 = local read "Vr2"() -> (w412:dbl)
                        n173 = local read "new_reactor_volume"() -> (w403:bool[])
                        n174 = for {
                          N: 5 -> [_]
                          tunnel: w403 -> [w417] mode=indexing
                          tunnel: [w414] -> w401 mode=indexing
                          n175 = Select(t=1.0, s=w417, f=0.0) -> (s? t:f=w414:dbl)
                        }
                        n176 = for {
                          N: 5 -> [_]
                          tunnel: w405 -> [w421] mode=indexing
                          tunnel: [w418] -> w404 mode=indexing
                          n177 = Select(t=1.0, s=w421, f=0.0) -> (s? t:f=w418:dbl)
                        }
                        n178 = script code="tube_diameters = [.01,.02,.03,.04];\naddpath('C:\\Users\\HPLC\\Dropbox (MIT)\\MoD Files\\MATLAB');\ncalculate_reactor_volumes;"("BayConfig"=w395, "Vr1"=w413, "Vr2"=w412, "Vr3"=w411, "Vr4"=w410, "Vr5"=w409, "tube_length"=w408, "tube_id"=w407, "new_len_react"=w404, "new_vol_react"=w401) -> ("Vr1"=w394:dbl, "Vr2"=w393:dbl, "Vr3"=w392:dbl, "Vr4"=w391:dbl, "Vr5"=w390:dbl)  [unwired: 1 in, 1 out]
                        n179 = local write "Vr1"(w394) -> ()
                        n180 = local write "Vr2"(w393) -> ()
                        n181 = local write "Vr3"(w392) -> ()
                        n182 = local write "Vr4"(w391) -> ()
                        n183 = local write "Vr5"(w390) -> ()
                      }
                      frame #4 {
                        n184 = local read "Setup Error"() -> (w424:bool)
                        n185 = case shown="True" w424 {
                          tunnel: [TRUE FALSE] -> w422
                          tunnel: ["" "Sytem setup has not been confirmed!"] -> w423
                          frame False {
                          }
                          frame True {
                            n186 = local read "Error Message"() -> (w429:string)
                            n187 = One Button Dialog(message=w429) -> ()  [unwired: 1 in, 1 out]
                          }
                        }
                        n188 = local write "System Confirm Not Clicked"(w423) -> ()
                        n189 = local write "Setup Confirm"(w422) -> ()
                      }
                    }
                  }
                }
              }
            }
            n190 = local read "Stop"() -> (w208:bool)
            n191 = Or(x=w209, y=w208) -> (x .or. y?=w207:bool)
            n192 = disable-structure shown="Disabled" {
              disable-tunnel: 400 -> [w215 _]
              frame Disabled {
                n193 = event shown="[1]" {
                  selector: _ -> [_ _]
                  dyn-events: _ -> [_ _]
                  timeout: w215 -> [_ _]
                  event Timeout {
                    n194 = event-data() -> ()  [unwired: 1 in, 3 out]
                  }
                  event #1 (no event record) {
                    n195 = event-data() -> ()  [unwired: 1 in, 6 out]
                    n196 = local read "Setup Confirm"() -> (w216:bool)
                    n197 = local read "Reaction Scheme Confirm"() -> (w217:bool)
                    n198 = Not(x=w216) -> (.not. x?=w219:bool)
                    n199 = And(x=w217, y=w219) -> (x .and. y?=w218:bool)
                    n200 = case shown="True" w218 {
                      frame False {
                      }
                      frame True {
                        w221 = u16 0 items=["                     Bypass", "                Hot Reactor", "                 Separator"] ("BAY 5")
                        w222 = u16 0 items=["                     Bypass", "                Hot Reactor", "                  Separator"] ("BAY 4")
                        w223 = u16 0 items=["                     Bypass", "                 Hot Reactor", "                  Separator"] ("BAY 3")
                        w224 = u16 0 items=["                     Bypass", "                Hot Reactor", "                  Separator"] ("BAY 2")
                        w225 = u16 0 items=["                 Bypass", "             Hot Reactor", "               Separator"] ("BAY 1")
                        n201 = local write "BAY 3"(w223) -> ()
                        n202 = local write "BAY 4"(w222) -> ()
                        n203 = local write "BAY 5"(w221) -> ()
                        n204 = local write "BAY 2"(w224) -> ()
                        n205 = local write "BAY 1"(w225) -> ()
                        n206 = local write "Synthesis Route Array"(string[][] [["3-Br-Pyridine _ Biphenyl", "K2CO3", "PhB(OH)2", "", "", ""]] ("Synthesis Route Array")) -> ()
                      }
                    }
                  }
                }
              }
              frame Enabled {
              }
            }
            n207 = disable-structure shown="Disabled" {
              disable-tunnel: 400 -> [w211 _]
              frame Disabled {
                n208 = event shown="[1]" {
                  selector: _ -> [_ _]
                  dyn-events: _ -> [_ _]
                  timeout: w211 -> [_ _]
                  event Timeout {
                    n209 = event-data() -> ()  [unwired: 1 in, 3 out]
                  }
                  event #1 (no event record) {
                    n210 = event-data() -> ()  [unwired: 1 in, 6 out]
                    n211 = call "File Dialog"("prompt"="Load previously saved xml file") -> ("selected path"=w213:path)  [unwired: 11 in, 3 out]
                    n212 = Path To String(path=w213) -> (string=w212:string)
                    n213 = script code="xmlDoc = xmlread(file_path);\nroot = xmlDoc.getDocumentElement();\nb = root.getChildNodes;\nrecipe = b.getElementsByTagName('Bay1').item(0);"("file_path"=w212) -> ()  [unwired: 1 in, 1 out]
                  }
                }
              }
              frame Enabled {
              }
            }
          }
        }
        frame #1 {
          n214 = local read "Stop"() -> (w431:bool)
          n215 = Not(x=w431) -> (.not. x?=w430:bool)
          n216 = case shown="True" w430 {
            tunnel: w432 -> [_ w435]
            frame False {
              "stop_button clicked" <- TRUE ("stop_button clicked")
            }
            frame True {
              # "Parameters Initilization"
              n217 = flat-sequence {
                tunnel: w435 -> [w437]
                tunnel: [w436] -> w434
                tunnel: w434 -> [w596]
                frame #0 {
                  # "Setup bays(RFID - verify)"
                  n218 = disable-structure shown="Disabled" {
                    frame Disabled {
                      n219 = local read "BAY 1"() -> ()  [unwired: 1 out]
                      n220 = local read "BAY 2"() -> ()  [unwired: 1 out]
                      n221 = local read "BAY 3"() -> ()  [unwired: 1 out]
                      n222 = local read "BAY 4"() -> ()  [unwired: 1 out]
                      n223 = local read "BAY 5"() -> ()  [unwired: 1 out]
                    }
                    frame Enabled {
                    }
                  }
                }
                frame #1 {
                  n224 = while {
                    tunnel: w437 -> [w440]
                    tunnel: [w439] -> w436
                    stop <- w443 stop-if-true
                    n225 = flat-sequence {
                      tunnel: [w457] -> w439
                      tunnel: w440 -> [w538]
                      tunnel: [w456] -> w438
                      frame #0 {
                        n226 = while {
                          stop <- w447 stop-if-true
                          n227 = event shown="[1] \"System Parameters Confirm Button\": Value Change" {
                            selector: _ -> [_ _]
                            dyn-events: _ -> [_ _]
                            timeout: u32 200 ("milliseconds to wait") -> [_ _]
                            tunnel: [FALSE TRUE] -> w445
                            event Timeout {
                              n228 = event-data() -> ()  [unwired: 1 in, 3 out]
                            }
                            event "System Parameters Confirm Button": Value Change {
                              n229 = event-data() -> ()  [unwired: 1 in, 5 out]
                              n230 = local write "System Parameters Confirm Button"(FALSE) -> ()
                            }
                          }
                          n231 = Wait (ms)(milliseconds to wait=u32 500) -> ()  [unwired: 1 out]
                          n232 = local read "Stop"() -> (w448:bool)
                          n233 = Or(x=w448, y=w445) -> (x .or. y?=w447:bool)
                        }
                      }
                      frame #1 {
                        w477 = 0 ("disabled index (col)")
                        w489 = 1 ("disabled index (col)")
                        # "Do while parameters have not been correctly entered"
                        n234 = local read "Bay Parameters"() -> (w476:T2)
                        n235 = local read "Synthesis Route Array"() -> (w490:string[][])
                        n236 = local read "Total Number of Experiments"() -> (w509:dbl)
                        n237 = Unbundle By Name(w476) -> ("Continue from previous optimization?"=w537:bool)
                        n238 = Unbundle By Name(w476) -> ("Excel File Name"=w539:string)
                        n239 = Unbundle By Name(w476) -> ("Matlab File"=w535:string)
                        n240 = Unbundle By Name(w476) -> ("Bay 1.Run at set flowrate"=w581:bool)
                        n241 = Unbundle By Name(w476) -> ("Bay 1.Pump 1 Flowrate"=w587:dbl)
                        n242 = Unbundle By Name(w476) -> ("Bay 1.Pump 2 Flowrate"=w586:dbl)
                        n243 = Unbundle By Name(w476) -> ("Bay 2.Run at set flowrate"=w579:bool)
                        n244 = Unbundle By Name(w476) -> ("Bay 2.Pump 3 Flowrate"=w585:dbl)
                        n245 = Unbundle By Name(w476) -> ("Bay 3.Pump 4 Flowrate"=w584:dbl)
                        n246 = Unbundle By Name(w476) -> ("Bay 3.Run at set flowrate"=w578:bool)
                        n247 = Unbundle By Name(w476) -> ("Bay 4.Run at set flowrate"=w575:bool)
                        n248 = Unbundle By Name(w476) -> ("Bay 4.Pump 5 Flowrate"=w583:dbl)
                        n249 = Unbundle By Name(w476) -> ("Bay 5.Pump 6 Flowrate"=w582:dbl)
                        n250 = Unbundle By Name(w476) -> ("Bay 5.Run at set flowrate"=w574:bool)
                        n251 = Index Array(array=w490, index (row)=3, index (col)=w489) -> (element=w483:string)
                        n252 = Index Array(array=w490, index (row)=2, index (col)=w489) -> (element=w481:string)
                        n253 = Index Array(array=w490, index (row)=1, index (col)=w489) -> (element=w479:string)
                        n254 = Index Array(array=w490, index (row)=0, index (col)=w489) -> (element=w492:string)
                        n255 = Index Array(array=w490, index (row)=4, index (col)=w489) -> (element=w485:string)
                        n256 = Index Array(array=w490, index (row)=5, index (col)=w489) -> (element=w487:string)
                        n257 = Build Array(w492, w479, w481, w483, w485, w487) -> (w493:string[])
                        n258 = Index Array(array=w490, index (row)=0 ("index"), index (col)=w477) -> (element=w515:string)
                        n259 = for {
                          tunnel: w493 -> [w589] mode=indexing
                          tunnel: [w588] -> w478 mode=indexing
                          n260 = script code="ctemp1 = str2num(c_temp);"("c_temp"=w589) -> ("ctemp1"=w588:dbl)  [unwired: 1 in, 1 out]
                        }
                        n261 = Boolean To (0,1)(Boolean=w579) -> (0, 1=w534:i16)
                        n262 = Boolean To (0,1)(Boolean=w575) -> (0, 1=w576:i16)
                        n263 = Boolean To (0,1)(Boolean=w578) -> (0, 1=w577:i16)
                        n264 = Boolean To (0,1)(Boolean=w537) -> (0, 1=w536:i16)
                        n265 = Boolean To (0,1)(Boolean=w581) -> (0, 1=w580:i16)
                        n266 = Boolean To (0,1)(Boolean=w574) -> (0, 1=w573:i16)
                        n267 = Index Array(array=w490, index (row)=1 ("index"), index (col)=w477) -> (element=w510:string)
                        n268 = Index Array(array=w490, index (row)=2 ("index"), index (col)=w477) -> (element=w511:string)
                        n269 = Unbundle By Name(w476) -> ("Bay 1.optimize_temp"=w572:bool)
                        n270 = Unbundle By Name(w476) -> ("Bay 1.optimize_tau"=w570:bool)
                        n271 = Unbundle By Name(w476) -> ("Bay 2.optimize_temp"=w568:bool)
                        n272 = Unbundle By Name(w476) -> ("Bay 2.optimize_tau"=w566:bool)
                        n273 = Unbundle By Name(w476) -> ("Bay 3.optimize_temp"=w564:bool)
                        n274 = Unbundle By Name(w476) -> ("Bay 3.optimize_tau"=w562:bool)
                        n275 = Unbundle By Name(w476) -> ("Bay 4.optimize_temp"=w560:bool)
                        n276 = Unbundle By Name(w476) -> ("Bay 4.optimize_tau"=w558:bool)
                        n277 = Index Array(array=w490, index (row)=3 ("index"), index (col)=w477) -> (element=w512:string)
                        n278 = Boolean To (0,1)(Boolean=w560) -> (0, 1=w559:i16)
                        n279 = Boolean To (0,1)(Boolean=w558) -> (0, 1=w557:i16)
                        n280 = Index Array(array=w490, index (row)=4 ("index"), index (col)=w477) -> (element=w513:string)
                        n281 = Boolean To (0,1)(Boolean=w562) -> (0, 1=w561:i16)
                        n282 = Boolean To (0,1)(Boolean=w568) -> (0, 1=w567:i16)
                        n283 = Boolean To (0,1)(Boolean=w572) -> (0, 1=w571:i16)
                        n284 = Boolean To (0,1)(Boolean=w566) -> (0, 1=w565:i16)
                        n285 = Boolean To (0,1)(Boolean=w570) -> (0, 1=w569:i16)
                        n286 = Boolean To (0,1)(Boolean=w564) -> (0, 1=w563:i16)
                        n287 = Unbundle By Name(w476) -> ("Bay 5.optimize_temp"=w556:bool)
                        n288 = Unbundle By Name(w476) -> ("Bay 5.optimize_tau"=w554:bool)
                        n289 = Index Array(array=w490, index (row)=5 ("index"), index (col)=w477) -> (element=w514:string)
                        n290 = Boolean To (0,1)(Boolean=w556) -> (0, 1=w555:i16)
                        n291 = Boolean To (0,1)(Boolean=w554) -> (0, 1=w553:i16)
                        n292 = Build Array(w571, w569, w567, w565, w563, w561, w559, w557, w555, w553) -> (w552:i16[])
                        n293 = Unbundle By Name(w476) -> ("Bay 1.Temperature Params"=w549:dbl[])
                        n294 = Unbundle By Name(w476) -> ("Bay 2.Temperature Params"=w548:dbl[])
                        n295 = Unbundle By Name(w476) -> ("Bay 2.Resisdence time params"=w543:dbl[])
                        n296 = Unbundle By Name(w476) -> ("Bay 3.Temperature Params"=w547:dbl[])
                        n297 = Unbundle By Name(w476) -> ("Bay 3.Resisdence time params"=w542:dbl[])
                        n298 = Unbundle By Name(w476) -> ("Bay 4.Temperature Params"=w546:dbl[])
                        n299 = Unbundle By Name(w476) -> ("Bay 4.Resisdence time params"=w541:dbl[])
                        n300 = Unbundle By Name(w476) -> ("Bay 5.Temperature Params"=w545:dbl[])
                        n301 = Unbundle By Name(w476) -> ("Bay 5.Resisdence time params"=w540:dbl[])
                        n302 = Unbundle By Name(w476) -> ("Bay 1.pump params 2"=w508:dbl[])
                        n303 = Unbundle By Name(w476) -> ("Bay 1.pump params 1"=w544:dbl[])
                        n304 = Unbundle By Name(w476) -> ("Bay 1.Run at set temperature"=w499:bool)
                        n305 = Unbundle By Name(w476) -> ("Bay 2.Run at set temperature"=w497:bool)
                        n306 = Unbundle By Name(w476) -> ("Bay 3.Run at set temperature"=w496:bool)
                        n307 = Unbundle By Name(w476) -> ("Bay 4.Run at set temperature"=w495:bool)
                        n308 = Unbundle By Name(w476) -> ("Bay 5.Run at set temperature"=w494:bool)
                        n309 = Unbundle By Name(w476) -> ("Bay 3.Temperature"=w505:dbl)
                        n310 = Unbundle By Name(w476) -> ("Bay 1.Temperature"=w507:dbl)
                        n311 = Unbundle By Name(w476) -> ("Bay 2.Temperature"=w506:dbl)
                        n312 = Unbundle By Name(w476) -> ("Bay 4.Temperature"=w504:dbl)
                        n313 = Unbundle By Name(w476) -> ("Bay 5.Temperature"=w503:dbl)
                        n314 = Unbundle By Name(w476) -> ("Bay 3.pump_num_ratio"=w528:dbl)
                        n315 = Unbundle By Name(w476) -> ("Bay 4.pump_num_ratio"=w525:dbl)
                        n316 = Unbundle By Name(w476) -> ("Bay 5.pump_num_ratio"=w522:dbl)
                        n317 = Unbundle By Name(w476) -> ("Bay 2.pump_num_ratio"=w531:dbl)
                        n318 = Unbundle By Name(w476) -> ("Bay 4.pump_at_ratio"=w527:bool)
                        n319 = Boolean To (0,1)(Boolean=w527) -> (0, 1=w526:i16)
                        n320 = Unbundle By Name(w476) -> ("Bay 3.pump_at_ratio"=w530:bool)
                        n321 = Boolean To (0,1)(Boolean=w530) -> (0, 1=w529:i16)
                        n322 = Unbundle By Name(w476) -> ("Bay 5.pump_at_ratio"=w524:bool)
                        n323 = Boolean To (0,1)(Boolean=w524) -> (0, 1=w523:i16)
                        n324 = Unbundle By Name(w476) -> ("Bay 2.pump_at_ratio"=w533:bool)
                        n325 = Boolean To (0,1)(Boolean=w533) -> (0, 1=w532:i16)
                        n326 = Build Array(w507, w506, w505, w504, w503) -> (w502:dbl[])
                        n327 = Build Array(w499, w497, w496, w495, w494) -> (w498:bool[])
                        n328 = local read "Syringe_pump?"() -> (w455:bool)
                        n329 = for {
                          N: 5 -> [_]
                          tunnel: w498 -> [w593] mode=indexing
                          tunnel: [w592] -> w500 mode=indexing
                          n330 = Select(t=1.0, s=w593, f=0.0) -> (s? t:f=w592:dbl)
                        }
                        n331 = Unbundle By Name(w476) -> ("Internal Standard?"=w467:bool)
                        n332 = Unbundle By Name(w476) -> ("increas_decrease_hplc_peak"=w468:bool)
                        n333 = Unbundle By Name(w476) -> ("Hplc Wait time(min)"=w460:dbl)
                        n334 = Unbundle By Name(w476) -> ("Total Number of Experiments 2"=w459:dbl)
                        n335 = Unbundle By Name(w476) -> ("hplc_start"=w464:dbl)
                        n336 = Unbundle By Name(w476) -> ("ISTD start"=w462:dbl)
                        n337 = Unbundle By Name(w476) -> ("hplc_end"=w463:dbl)
                        n338 = Unbundle By Name(w476) -> ("throughput_yield"=w469:bool)
                        n339 = Unbundle By Name(w476) -> ("ISTD end"=w461:dbl)
                        n340 = Select(t=1.0, s=w455, f=0.0) -> (s? t:f=w454:dbl)
                        n341 = Select(t=1.0, s=w468, f=0.0) -> (s? t:f=w466:dbl)
                        n342 = Select(t=1.0, s=w467, f=0.0) -> (s? t:f=w465:dbl)
                        n343 = Select(t=0.0, s=w469, f=1.0) -> (s? t:f=w458:dbl)
                        n344 = script code="system_error = 0;\nnumPeaks = 1;\nstart_phase_time = 1;\nis_redo_exp = 0;\nFvalues = [];\nHPLC_Area = [];\n\nT1_span = [1 1]; T2_span = [1 1]; T3_span = [1 1]; T4_span = [1 1]; T5_span = [1 1];\nT_span = [T1_span;T2_span;T3_span;T4_span;T5_span];\n p1_span =  [1 1]; p2_span =  [1 1]; p3_span =  [1 1]; p4_span =  [1 1]; p5_span =  [1 1];  p6_span =  [1 1];\nOpt_params = [0 0 0 0 0 0 0 0 0 0 0];\nT_params = [T1_params;T2_params;T3_params;T4_params;T5_params];\npump_params = [pump1_params;pump2_params;pump3_params;pump4_params;pump5_params;pump6_params];\nopt_ctr = 0;ncall = 100;record_data = true;\nT1_SP = 23; T2_SP = 23; T3_SP = 23; T4_SP = 23; T5_SP = 23;\nT_span = [T1_span;T2_span;T3_span;T4_span;T5_span];\np_span = [p1_span;p2_span;p3_span;p4_span;p5_span;p6_span];\nno_errors = 1;\nP1 = 0; P2 =0; P3 = 0; P4 = 0; P5 = 0; P6 = 0;\nP = [P1, P2, P3,P4, P5, P6];\nis_first_set_of_exp = true;\nerror_message = 'System has no errors to report';\naddpath(genpath('C:\\Users\\HPLC\\Dropbox (MIT)\\MoD Files\\MATLAB'))\n%addpath(genpath('C:\\Users\\Admin\\Dropbox (MIT)\\MoD Files\\MATLAB'))\nallMSData = [];allHPLCData = [];allHPLCFile = [];\nBay_ratio = [0,Bay2_ratio,Bay3_ratio,Bay4_ratio,Bay5_ratio];\nBay_pump_ratio = [1, Bay2_pump_ratio, Bay3_pump_ratio, Bay4_pump_ratio, Bay5_pump_ratio];\nP_setrate = [P1_setrate, P2_setrate, P3_setrate, P4_setrate, P5_setrate, P6_setrate];\nuse_flowrate = [use_flowrate1, use_flowrate2,use_flowrate3, use_flowrate4, use_flowrate5];\npump_chem_name= []\nCurrExp = 1;\n% ****************************************************************************************************\n%Setup optimization\n   setup_optimization_params;\n   initialize_opt = 0;\n   nstop0 = 0;\n%*****************************************************************************************************\n% Setup excel and xml file writing\npath(path, pa);\nnumMSSig = 1;\nsetup_excel_output;\n%***************************************************************************************************\nredo = false;\nncall = ncall_in;"("use_flowrate1"=w580, "P1_setrate"=w587, "P2_setrate"=w586, "P3_setrate"=w585, "P4_setrate"=w584, "P5_setrate"=w583, "P6_setrate"=w582, "use_flowrate2"=w534, "use_flowrate3"=w577, "use_flowrate4"=w576, "use_flowrate5"=w573, "Optimize_params"=w552, "T1_params"=w549, "T2_params"=w548, "T3_params"=w547, "T4_params"=w546, "T5_params"=w545, "pump1_params"=w544, "pump3_params"=w543, "pump4_params"=w542, "pump5_params"=w541, "pump6_params"=w540, "xl_file"=w539, "pa"=w538, "Continue"=w536, "matlabsavefile"=w535, "Bay2_ratio"=w532, "Bay2_pump_ratio"=w531, "Bay3_ratio"=w529, "Bay3_pump_ratio"=w528, "Bay4_ratio"=w526, "Bay4_pump_ratio"=w525, "Bay5_ratio"=w523, "Bay5_pump_ratio"=w522, "pump1_chem"=w515, "pump6_chem"=w514, "pump5_chem"=w513, "pump4_chem"=w512, "pump3_chem"=w511, "pump2_chem"=w510, "Pump_concen"=w478, "ncall_in"=w509, "pump2_params"=w508, "T_SP"=w502, "Run_at_T_SP"=w500, "dcr_hplc_peak"=w466, "use_internal_std"=w465, "hplc_peak_start"=w464, "hplc_peak_end"=w463, "ISTD_start"=w462, "ISTD_end"=w461, "hplc_wait_time"=w460, "tot_num_exp"=w459, "throughput_yield"=w458, "syringe_pump"=w454) -> ("no_errors"=w551:dbl, "error_message"=w550:string)  [unwired: 1 in, 1 out]
                        n345 = Not Equal To 0?(x=w551) -> (x != 0?=w456:bool)
                        n346 = Not(x=w456) -> (.not. x?=w457:bool)
                        n347 = case shown="False" w457 {
                          tunnel: w550 -> [_ w595]
                          frame False {
                            n348 = local write "Setup Confirm 2"(TRUE ("Setup Confirm 2")) -> ()
                          }
                          frame True {
                            n349 = One Button Dialog(message=w595) -> ()  [unwired: 1 in, 1 out]
                          }
                        }
                      }
                    }
                    n350 = local read "Stop"() -> (w442:bool)
                    n351 = Or(x=w438, y=w442) -> (x .or. y?=w443:bool)
                    n352 = Wait (ms)(milliseconds to wait=u32 500) -> ()  [unwired: 1 out]
                  }
                }
                frame #2 {
                  n353 = local write "System Error"(w596) -> ()
                }
              }
            }
          }
        }
        frame #2 {
          # "Run Initial diagnostics"
        }
        frame #3 {
          # "Run System"
          n354 = while {
            tunnel: w597 -> [w1329]
            stop <- w1333 stop-if-true
            n355 = local read "running?"() -> (w1328:bool)
            n356 = local read "Temperature Control 1"() -> (w1330:bool)
            n357 = And(x=w1328, y=w1330) -> (x .and. y?=w1331:bool)
            n358 = case shown="True" w1331 {
              tunnel: w1329 -> [_ w1335]
              frame False {
                n359 = local write "Temp SS? 1"(TRUE ("Temp SS? 1")) -> ()
              }
              frame True {
                # "Bay 1 Temperature Controller"
                n360 = local read "Temperature SP 1"() -> (w1336:dbl)
                n361 = local read "Temperature 1"() -> (w1340:dbl)
                n362 = local read "SSR Duration 1"() -> (w1355:dbl)
                n363 = call-poly <vilib>:"PID Online Autotuning.vi"("setpoint"=w1336, "manipulated variable"=w1355, "autotuning parameters"=T9 {"type of controller"=enum."PID", "relay cycles"=3, "relay amplitude"=1.0, "control specifications"=enum."Normal", "PV noise level"=0.1} ("Autotuning Parameters R1"), "process variable"=w1340, "PID gains in"=T8 {"Proportional gain Kc"=0.38538, "Integral time Ti (sec)"=0.524375, "Derivative time Ti (sec)"=0.12585} ("PID gains 2")) -> ("setpoint out"=w1361:dbl, "process variable out"=w1360:dbl, "PID gains out"=w1357:T17)  [unwired: 6 in, 2 out]
                n364 = call <vilib>:"PID Autotuning (Temperature).vi"("desired temperature"=w1361, "measured temperature"=w1360, "plant parameters in"=w1357, "output range"=cluster{"output high":dbl, "output low":dbl} {"output high"=3.0, "output low"=-1.0} ("Output range")) -> ("output"=w1353:dbl)  [unwired: 12 in, 3 out]
                n365 = local write "SSR Duration 1"(w1353) -> ()
                n366 = Subtract(x=w1336, y=w1340) -> (x-y=w1347:dbl)
                n367 = Absolute Value(x=w1347) -> (abs(x)=w1350:dbl)
                n368 = Multiply(x=1000.0, y=w1353) -> (x*y=w1351:dbl)
                n369 = Greater Than 0?(x=w1351) -> (x > 0?=w1345:bool)
                n370 = Less Or Equal?(x=w1350, y=1.2) -> (x <= y?=w1348:bool)
                n371 = Greater?(x=w1336, y=w1340) -> (0:w1346:bool)
                n372 = And(x=w1345, y=w1346) -> (x .and. y?=w1343:bool)
                n373 = local write "Temp SS? 1"(w1348) -> ()
                n374 = Subtract(x=w1340, y=10.0) -> (x-y=w1341:dbl)
                n375 = Less?(x=w1341, y=w1336) -> (x < y?=w1344:bool)
                n376 = And(x=w1344, y=w1343) -> (x .and. y?=w1342:bool)
                n377 = case shown="True" w1342 {
                  tunnel: [errorcluster {"status"=FALSE, "code"=0, "source"=""} ("error out") w1371] -> _
                  tunnel: 2 -> [_ w1368]
                  tunnel: w1351 -> [w1365 w1369]
                  tunnel: [0.0 w1373] -> w1338
                  tunnel: w1336 -> [_ w1372]
                  tunnel: w1335 -> [_ w1370]
                  frame False {
                    n378 = Absolute Value(x=w1365) -> (abs(x)=w1366:dbl)
                    n379 = Wait (ms)(milliseconds to wait=w1366) -> ()  [unwired: 1 out]
                  }
                  frame True {
                    n380 = call "TurnOnRelayArduino.vi"("channel"=w1368, "duration"=w1369, "LINX Resource"=w1370) -> ("error out"=w1371:errorcluster)  [unwired: 7 in, 1 out]
                    n381 = script code="tempdiff1= SP1 - T1;\nif tempdiff1 > 10\n  if slope1 < .01\n     temp_check1 = temp_check1 + 1;\n  else\n      temp_check1 =0;\n  end\nend\n\nif temp_check1 > 9\n  temp_error1 = 1\nend"("SP1"=w1372) -> ("temp_error1"=w1373:dbl)  [unwired: 1 in, 1 out]
                  }
                }
                n382 = Not Equal To 0?(x=w1338) -> (x != 0?=w1337:bool)
                n383 = case shown="True" w1337 {
                  frame False {
                  }
                  frame True {
                    n384 = local write "Error Message"("Bay 1 Temperature Heating Error") -> ()
                  }
                }
                n385 = case shown="True" w1337 {
                  tunnel: w1337 -> [_ w1363]
                  frame False {
                  }
                  frame True {
                    n386 = local write "System Error"(w1363) -> ()
                    n387 = local write "Stop"(w1363) -> ()
                  }
                }
              }
            }
            n388 = Wait (ms)(milliseconds to wait=u32 400) -> ()  [unwired: 1 out]
            n389 = local read "Stop"() -> (w1333:bool)
          }
          n390 = local read "Bay Parameters"() -> (w601:T2)
          n391 = while {
            tunnel: w597 -> [w1283]
            stop <- w1287 stop-if-true
            n392 = local read "running?"() -> (w1282:bool)
            n393 = local read "Temperature Control 2"() -> (w1284:bool)
            n394 = And(x=w1282, y=w1284) -> (x .and. y?=w1285:bool)
            n395 = case shown="True" w1285 {
              tunnel: w1283 -> [_ w1289]
              frame False {
                n396 = local write "Temp SS? 2"(TRUE ("Temp SS? 2")) -> ()
              }
              frame True {
                # "Bay 2 Temperature Controller"
                n397 = local read "Temperature SP 2"() -> (w1291:dbl)
                n398 = local read "Temperature 2"() -> (w1294:dbl)
                n399 = local read "SSR Duration 2"() -> (w1312:dbl)
                n400 = call-poly <vilib>:"PID Online Autotuning.vi"("setpoint"=w1291, "manipulated variable"=w1312, "autotuning parameters"=T9 {"type of controller"=enum."PID", "relay cycles"=3, "relay amplitude"=1.0, "control specifications"=enum."Normal", "PV noise level"=0.1} ("Autotuning Parameters R1"), "process variable"=w1294, "PID gains in"=T8 {"Proportional gain Kc"=0.38538, "Integral time Ti (sec)"=0.524375, "Derivative time Ti (sec)"=0.12585} ("PID gains 2")) -> ("setpoint out"=w1310:dbl, "process variable out"=w1309:dbl, "PID gains out"=w1315:T17)  [unwired: 6 in, 2 out]
                n401 = call <vilib>:"PID Autotuning (Temperature).vi"("desired temperature"=w1310, "measured temperature"=w1309, "plant parameters in"=w1315, "output range"=cluster{"output high":dbl, "output low":dbl} {"output high"=3.0, "output low"=-1.0} ("Output range")) -> ("output"=w1305:dbl)  [unwired: 12 in, 3 out]
                n402 = local write "SSR Duration 2"(w1305) -> ()
                n403 = Greater?(x=w1291, y=w1294) -> (0:w1300:bool)
                n404 = Multiply(x=1000.0, y=w1305) -> (x*y=w1307:dbl)
                n405 = Greater Than 0?(x=w1307) -> (x > 0?=w1299:bool)
                n406 = And(x=w1299, y=w1300) -> (x .and. y?=w1297:bool)
                n407 = Subtract(x=w1291, y=w1294) -> (x-y=w1302:dbl)
                n408 = Absolute Value(x=w1302) -> (abs(x)=w1304:dbl)
                n409 = Subtract(x=w1294, y=10.0) -> (x-y=w1296:dbl)
                n410 = Less Or Equal?(x=w1304, y=1.2) -> (x <= y?=w1301:bool)
                n411 = local write "Temp SS? 2"(w1301) -> ()
                n412 = Less?(x=w1296, y=w1291) -> (x < y?=w1298:bool)
                n413 = And(x=w1298, y=w1297) -> (x .and. y?=w1293:bool)
                n414 = case shown="True" w1293 {
                  tunnel: [errorcluster {"status"=FALSE, "code"=0, "source"=""} ("error out") w1325] -> _
                  tunnel: 3 -> [_ w1322]
                  tunnel: w1307 -> [w1319 w1323]
                  tunnel: [0.0 w1327] -> w1292
                  tunnel: w1291 -> [_ w1326]
                  tunnel: w1289 -> [_ w1324]
                  frame False {
                    n415 = Absolute Value(x=w1319) -> (abs(x)=w1320:dbl)
                    n416 = Wait (ms)(milliseconds to wait=w1320) -> ()  [unwired: 1 out]
                  }
                  frame True {
                    n417 = call "TurnOnRelayArduino.vi"("channel"=w1322, "duration"=w1323, "LINX Resource"=w1324) -> ("error out"=w1325:errorcluster)  [unwired: 7 in, 1 out]
                    n418 = script code="tempdiff2= SP2 - T2;\nif tempdiff2 > 10\n  if slope2 < .01\n     temp_check2 = temp_check2 + 1;\n  else\n      temp_check2 =0;\n  end\nend\n\nif temp_check2 > 9\n  temp_error2 = 1\nend"("SP2"=w1326) -> ("temp_error2"=w1327:dbl)  [unwired: 1 in, 1 out]
                  }
                }
                n419 = Not Equal To 0?(x=w1292) -> (x != 0?=w1290:bool)
                n420 = case shown="True" w1290 {
                  frame False {
                  }
                  frame True {
                    n421 = local write "Error Message"("Bay 2 Temperature Heating Error") -> ()
                  }
                }
                n422 = case shown="True" w1290 {
                  tunnel: w1290 -> [_ w1317]
                  frame False {
                  }
                  frame True {
                    n423 = local write "Stop"(w1317) -> ()
                    n424 = local write "System Error"(w1317) -> ()
                  }
                }
              }
            }
            n425 = local read "Stop"() -> (w1287:bool)
            n426 = Wait (ms)(milliseconds to wait=u32 400) -> ()  [unwired: 1 out]
          }
          n427 = local read "Stop"() -> (w598:bool)
          n428 = Not(x=w598) -> (.not. x?=w600:bool)
          n429 = case shown="True" w600 {
            tunnel: w601 -> [_ w606]
            tunnel: w599 -> [_ w605]
            tunnel: w597 -> [_ w604]
            frame False {
            }
            frame True {
              n430 = while {
                tunnel: w606 -> [w620]
                tunnel: w605 -> [w612]
                tunnel: w604 -> [w607]
                i -> [w619]
                stop <- w613 stop-if-true
                n431 = local read "running?"() -> (w608:bool)
                n432 = Wait (ms)(milliseconds to wait=u32 1000) -> ()  [unwired: 1 out]
                n433 = Increment(x=w619) -> (x+1=w609:i32)
                n434 = case shown="True" w608 {
                  tunnel: w619 -> [w625 _]
                  tunnel: w620 -> [_ _]
                  tunnel: [w627 w631] -> w610
                  tunnel: [0.0 w632] -> w615
                  tunnel: w612 -> [_ w630]
                  tunnel: w607 -> [_ w628]
                  frame False {
                    # "STANDBY MODE"
                    n435 = Add(x=w625, y=2.0) -> (x+y=w627:dbl)
                  }
                  frame True {
                    n436 = flat-sequence {
                      tunnel: w630 -> [w634]
                      tunnel: [w634] -> w629
                      tunnel: [w646] -> w632
                      tunnel: [200.0] -> w631
                      tunnel: w629 -> [w644]
                      tunnel: w628 -> [w635]
                      frame #0 {
                        n437 = local write "stop_xl_write"(FALSE ("stop_xl_write")) -> ()
                      }
                      frame #1 {
                        # "Increase flowrate of dilution stream"
                        # "Wait mixed stream reaches SL"
                        # "SNOBFIT"
                        # "Optimize"
                        # "Run Experimental Conditions"
                        # "Optimize/Synthesize"
                        n438 = local read "Syringe_pump?"() -> (w638:bool)
                        n439 = local read "Stop"() -> (w641:bool)
                        n440 = Not(x=w641) -> (.not. x?=w640:bool)
                        n441 = case shown="True" w640 {
                          tunnel: [1.0 w668] -> w649
                          tunnel: [w656 w667] -> w643
                          tunnel: [0.0 w666] -> w642
                          tunnel: [w656 w665] -> w639
                          tunnel: w638 -> [_ w662]
                          frame False {
                            w656 = dbl[] []
                          }
                          frame True {
                            n442 = Select(t=1.0, s=w662, f=0.0) -> (s? t:f=w661:dbl)
                            n443 = script code="optimization_main_loop"("syringe_pump"=w661) -> ("Conditions_Array"=w667:dbl[], "opt_ctr"=w668:dbl, "P_tot"=w666:dbl, "tau_array"=w665:dbl[], "experiment_history"=w663:dbl[][])  [unwired: 1 in, 1 out]
                            n444 = call-poly <vilib>:"Array To Matrix.vi"("Real 2D Array"=w663) -> ("Real Matrix"=w664:T18)
                            n445 = local write "experiment history"(w664) -> ()
                          }
                        }
                        "P_tot" <- w642
                        n446 = local read "COMM Port :: Milligat Pumps"() -> (w650:refnum<visa-resource-name>)
                        n447 = Equal?(x=w649, y=1.0) -> (x = y?=w647:bool)
                        n448 = flat-sequence {
                          tunnel: w643 -> [w1127]
                          tunnel: w639 -> [w1121]
                          frame #0 {
                            # "Start recording data"
                            n449 = Index Array(array=w1127, index=5) -> (element=w1139:dbl)
                            n450 = Index Array(array=w1127, index=0) -> (element=w1134:dbl)
                            n451 = Index Array(array=w1127, index=1) -> (element=w1135:dbl)
                            n452 = Index Array(array=w1127, index=2) -> (element=w1137:dbl)
                            n453 = Index Array(array=w1127, index=3) -> (element=w1136:dbl)
                            n454 = Index Array(array=w1127, index=4) -> (element=w1138:dbl)
                            n455 = local write "Pump setpoint(ul/min) 2"(w1135) -> ()
                            n456 = local write "Pump setpoint(ul/min) 4"(w1137) -> ()
                            n457 = local write "Pump setpoint(ul/min) 5"(w1138) -> ()
                            n458 = local write "Pump setpoint(ul/min) 3"(w1136) -> ()
                            n459 = local write "Pump setpoint(ul/min) 6"(w1139) -> ()
                            n460 = local write "Pump setpoint(ul/min) 1"(w1134) -> ()
                            n461 = Index Array(array=w1121, index=0) -> (element=w1126:dbl)
                            n462 = Index Array(array=w1121, index=4) -> (element=w1125:dbl)
                            n463 = Index Array(array=w1121, index=3) -> (element=w1124:dbl)
                            n464 = Index Array(array=w1121, index=2) -> (element=w1123:dbl)
                            n465 = Index Array(array=w1121, index=1) -> (element=w1122:dbl)
                            n466 = local write "tau 2"(w1122) -> ()
                            n467 = local write "tau 3"(w1123) -> ()
                            n468 = local write "tau 4"(w1124) -> ()
                            n469 = local write "tau 5"(w1125) -> ()
                            n470 = local write "tau 1"(w1126) -> ()
                          }
                        }
                        n471 = flat-sequence {
                          tunnel: w650 -> [w672]
                          tunnel: w643 -> [w671]
                          tunnel: w647 -> [w670]
                          tunnel: [w670] -> w655
                          tunnel: w644 -> [w669]
                          tunnel: w655 -> [w824]
                          tunnel: [w824] -> w654
                          tunnel: w654 -> [w844]
                          tunnel: [w842] -> w637
                          tunnel: w637 -> [w867]
                          tunnel: [w867] -> w636
                          tunnel: w635 -> [w866]
                          tunnel: w643 -> [w885]
                          tunnel: w636 -> [w884]
                          tunnel: w635 -> [w883]
                          tunnel: [w1057] -> w653
                          tunnel: w653 -> [w1070]
                          tunnel: [w1070] -> w652
                          tunnel: w652 -> [w1078]
                          tunnel: [w1078] -> w651
                          tunnel: [w1115] -> w646
                          tunnel: w651 -> [w1115]
                          frame #0 {
                            # "Setup pump flowrates and temperature setpoints"
                            n472 = stacked-sequence {
                              tunnel: w672 -> [w695 _ _ _ _]
                              tunnel: w672 -> [_ w736 _ _ _]
                              tunnel: w672 -> [_ _ w764 _ _]
                              tunnel: w672 -> [_ _ _ w789 _]
                              tunnel: w672 -> [_ _ _ _ w814]
                              tunnel: w671 -> [w692 w734 w762 w787 w811]
                              tunnel: w670 -> [w682 w727 w757 w780 w805]
                              tunnel: w669 -> [w680 _ _ _ _]
                              frame #0 {
                                # "Bay 1"
                                n473 = local read "Syringe_pump?"() -> (w681:bool)
                                n474 = Index Array(array=w692, index=0) -> (element=w690:dbl)
                                n475 = local read "BAY 1"() -> (w675:u16)
                                n476 = Index Array(array=w692, index=1) -> (element=w689:dbl)
                                n477 = Index Array(array=w692, index=6) -> (element=w688:dbl)
                                n478 = script code="MATLAB script"("T1_SP"=w688) -> ()  [unwired: 1 in, 1 out]
                                n479 = Less Or Equal?(x=w675, y=u16 4) -> (x <= y?=w677:bool)
                                n480 = Greater Or Equal?(x=w675, y=u16 1) -> (x >= y?=w678:bool)
                                n481 = And(x=w678, y=w677) -> (x .and. y?=w679:bool)
                                n482 = Greater Than 0?(x=w690) -> (x > 0?=w687:bool)
                                n483 = And(x=w687, y=w682) -> (x .and. y?=w686:bool)
                                n484 = Greater Than 0?(x=w689) -> (x > 0?=w685:bool)
                                n485 = Wait (ms)(milliseconds to wait=u32 300) -> ()  [unwired: 1 out]
                                n486 = And(x=w685, y=w682) -> (x .and. y?=w684:bool)
                                n487 = And(x=w679, y=w682) -> (x .and. y?=w683:bool)
                                n488 = case shown="False" w681 {
                                tunnel: w695 -> [w698 _]
                                tunnel: w689 -> [w697 w703]
                                tunnel: w684 -> [w696 w704]
                                tunnel: w680 -> [_ w702]
                                frame False {
                                n489 = case shown="False" w696 {
                                tunnel: w698 -> [w700 _]
                                tunnel: w697 -> [w699 _]
                                frame False {
                                n490 = call "PumpDispense.vi"("Flowrate(ul/min)"=w699, "Pump Address"="j", "Pump COMM Port"=w700) -> ()  [unwired: 7 in, 2 out]
                                }
                                frame True {
                                }
                                }
                                }
                                frame True {
                                n491 = case shown="False" w704 {
                                tunnel: w703 -> [_ w706]
                                tunnel: w702 -> [w705 w707]
                                frame False {
                                n492 = call <instrlib>:"Stop Pump.vi"("VISA resource name"=w705) -> ()  [unwired: 9 in, 2 out]
                                }
                                frame True {
                                w708 = u16 0 items=["Infuse", "Withdraw"] ("Run Direction (0:Infuse)")
                                w709 = u32 4 items=["milliliters per hour (ml/hr)", "milliliters per minute (ml/min)", "milliliters per second (ml/sec)", "microliters per hour (ul/hr)", "microliters per minute (ul/min)", "microliters per second (ul/sec)", "nanoliters per hour (nl/hr)", "nanoliters per minute (nl/min)", "nanoliters per second (nl/sec)", "picoliters per hour (pl/hr)", "picoliters per minute (pl/min)", "picoliters per second (pl/sec)"] ("Flow Rate Units (1:ml/min)")
                                w710 = u16 0 items=["Infuse", "Withdraw"] ("Pump Direction (0:Infuse)")
                                n493 = call <instrlib>:"Configure Flow Rate & Direction.vi"("VISA resource name"=w707, "Pump Direction (0:Infuse)"=w710, "Flow Rate (5.00)"=w706, "Flow Rate Units (1:ml/min)"=w709) -> ("VISA resource name out"=w711:refnum<visa-resource-name>)  [unwired: 10 in, 1 out]
                                n494 = call <instrlib>:"Start Pump.vi"("Run Direction (0:Infuse)"=w708, "VISA resource name"=w711) -> ()  [unwired: 8 in, 2 out]
                                }
                                }
                                }
                                }
                                n495 = case shown="False" w686 {
                                tunnel: w695 -> [w715 w717]
                                tunnel: w690 -> [_ w718]
                                frame False {
                                n496 = call "PumpStop.vi"("Pump Address"="f", "Pump COMM Port"=w715) -> ()  [unwired: 9 in, 1 out]
                                }
                                frame True {
                                n497 = call "PumpDispense.vi"("Flowrate(ul/min)"=w718, "Pump Address"="f", "Pump COMM Port"=w717) -> ()  [unwired: 7 in, 2 out]
                                }
                                }
                                n498 = case shown="True" w683 {
                                tunnel: w688 -> [_ w714]
                                frame False {
                                n499 = local write "Temperature Control 1"(FALSE) -> ()
                                }
                                frame True {
                                n500 = local write "Temperature SP 1"(w714) -> ()
                                n501 = local write "Temperature Control 1"(TRUE ("Temperature Control 1")) -> ()
                                }
                                }
                              }
                              frame #1 {
                                # "Bay 2"
                                n502 = local read "BAY 2"() -> (w723:u16)
                                n503 = Index Array(array=w734, index=2) -> (element=w731:dbl)
                                n504 = Index Array(array=w734, index=7) -> (element=w732:dbl)
                                n505 = script code="MATLAB script"("T2_SP"=w732) -> ()  [unwired: 1 in, 1 out]
                                n506 = Greater Than 0?(x=w731) -> (x > 0?=w729:bool)
                                n507 = And(x=w729, y=w727) -> (x .and. y?=w728:bool)
                                n508 = Greater Or Equal?(x=w723, y=u16 1) -> (x >= y?=w721:bool)
                                n509 = Less Or Equal?(x=w723, y=u16 4) -> (x <= y?=w726:bool)
                                n510 = And(x=w721, y=w726) -> (x .and. y?=w725:bool)
                                n511 = And(x=w725, y=w727) -> (x .and. y?=w730:bool)
                                n512 = case shown="True" w730 {
                                tunnel: w732 -> [_ w743]
                                frame False {
                                n513 = local write "Temperature Control 2"(FALSE) -> ()
                                }
                                frame True {
                                n514 = local write "Temperature Control 2"(TRUE ("Temperature Control 2")) -> ()
                                n515 = local write "Temperature SP 2"(w743) -> ()
                                }
                                }
                                n516 = case shown="False" w728 {
                                tunnel: w731 -> [_ w739]
                                tunnel: w736 -> [w737 w740]
                                frame False {
                                n517 = call "PumpStop.vi"("Pump Address"="i", "Pump COMM Port"=w737) -> ()  [unwired: 9 in, 1 out]
                                }
                                frame True {
                                n518 = call "PumpDispense.vi"("Flowrate(ul/min)"=w739, "Pump Address"="i", "Pump COMM Port"=w740) -> ()  [unwired: 7 in, 2 out]
                                }
                                }
                                n519 = Wait (ms)(milliseconds to wait=u32 300) -> ()  [unwired: 1 out]
                              }
                              frame #2 {
                                # "Bay 3"
                                n520 = local read "BAY 3"() -> (w752:u16)
                                n521 = Index Array(array=w762, index=3) -> (element=w760:dbl)
                                n522 = Not Equal To 0?(x=w760) -> (x != 0?=w759:bool)
                                n523 = Index Array(array=w762, index=8) -> (element=w747:dbl)
                                n524 = script code="MATLAB script"("T3_SP"=w747) -> ()  [unwired: 1 in, 1 out]
                                n525 = Less Or Equal?(x=w752, y=u16 4) -> (x <= y?=w756:bool)
                                n526 = Greater Or Equal?(x=w752, y=u16 1) -> (x >= y?=w753:bool)
                                n527 = And(x=w753, y=w756) -> (x .and. y?=w751:bool)
                                n528 = And(x=w751, y=w757) -> (x .and. y?=w749:bool)
                                n529 = And(x=w759, y=w757) -> (x .and. y?=w758:bool)
                                n530 = Not Equal?(x=w747, y=23.0) -> (x != y?=w748:bool)
                                n531 = And(x=w749, y=w748) -> (x .and. y?=w745:bool)
                                n532 = case shown="False" w758 {
                                tunnel: w760 -> [_ w767]
                                tunnel: w764 -> [w765 w768]
                                frame False {
                                n533 = call "PumpStop.vi"("Pump Address"="g", "Pump COMM Port"=w765) -> ()  [unwired: 9 in, 1 out]
                                }
                                frame True {
                                n534 = call "PumpDispense.vi"("Flowrate(ul/min)"=w767, "Pump Address"="g", "Pump COMM Port"=w768) -> ()  [unwired: 7 in, 2 out]
                                }
                                }
                                n535 = case shown="True" w745 {
                                tunnel: w747 -> [_ w771]
                                frame False {
                                n536 = local write "Temperature Control 3"(FALSE) -> ()
                                }
                                frame True {
                                n537 = local write "Temperature Control 3"(TRUE ("Temperature Control 3")) -> ()
                                n538 = local write "Temperature SP 3"(w771) -> ()
                                }
                                }
                                n539 = Wait (ms)(milliseconds to wait=u32 300) -> ()  [unwired: 1 out]
                              }
                              frame #3 {
                                # "Bay 4"
                                n540 = Index Array(array=w787, index=9) -> (element=w784:dbl)
                                n541 = script code="MATLAB script"("T4_SP"=w784) -> ()  [unwired: 1 in, 1 out]
                                n542 = Index Array(array=w787, index=4) -> (element=w785:dbl)
                                n543 = Not Equal To 0?(x=w785) -> (x != 0?=w783:bool)
                                n544 = local read "BAY 4"() -> (w774:u16)
                                n545 = And(x=w783, y=w780) -> (x .and. y?=w782:bool)
                                n546 = Less Or Equal?(x=w774, y=u16 4) -> (x <= y?=w779:bool)
                                n547 = Greater Or Equal?(x=w774, y=u16 1) -> (x >= y?=w776:bool)
                                n548 = And(x=w776, y=w779) -> (x .and. y?=w775:bool)
                                n549 = And(x=w775, y=w780) -> (x .and. y?=w781:bool)
                                n550 = case shown="True" w782 {
                                tunnel: w789 -> [w790 w793]
                                tunnel: w785 -> [_ w792]
                                frame False {
                                n551 = call "PumpStop.vi"("Pump Address"="e", "Pump COMM Port"=w790) -> ()  [unwired: 9 in, 1 out]
                                }
                                frame True {
                                n552 = call "PumpDispense.vi"("Flowrate(ul/min)"=w792, "Pump Address"="e", "Pump COMM Port"=w793) -> ()  [unwired: 7 in, 2 out]
                                }
                                }
                                n553 = case shown="True" w781 {
                                tunnel: w784 -> [_ w796]
                                frame False {
                                n554 = local write "Temperature Control 4"(FALSE ("Temperature Control 4")) -> ()
                                }
                                frame True {
                                n555 = local write "Temperature SP 4"(w796) -> ()
                                n556 = local write "Temperature Control 4"(TRUE ("Temperature Control 5")) -> ()
                                }
                                }
                                n557 = Wait (ms)(milliseconds to wait=u32 300) -> ()  [unwired: 1 out]
                              }
                              frame #4 {
                                # "Bay 5"
                                n558 = Index Array(array=w811, index=5) -> (element=w809:dbl)
                                n559 = Index Array(array=w811, index=4) -> (element=w810:dbl)
                                n560 = script code="MATLAB script"("T5_SP"=w810) -> ()  [unwired: 1 in, 1 out]
                                n561 = local read "BAY 5"() -> (w800:u16)
                                n562 = Not Equal To 0?(x=w809) -> (x != 0?=w807:bool)
                                n563 = And(x=w807, y=w805) -> (x .and. y?=w806:bool)
                                n564 = Less Or Equal?(x=w800, y=u16 4) -> (x <= y?=w804:bool)
                                n565 = Greater Or Equal?(x=w800, y=u16 1) -> (x >= y?=w801:bool)
                                n566 = case shown="False" w806 {
                                tunnel: w814 -> [w815 w818]
                                tunnel: w809 -> [_ w817]
                                frame False {
                                n567 = call "PumpStop.vi"("Pump Address"="h", "Pump COMM Port"=w815) -> ()  [unwired: 9 in, 1 out]
                                }
                                frame True {
                                n568 = call "PumpDispense.vi"("Flowrate(ul/min)"=w817, "Pump Address"="h", "Pump COMM Port"=w818) -> ()  [unwired: 7 in, 2 out]
                                }
                                }
                                n569 = And(x=w801, y=w804) -> (x .and. y?=w799:bool)
                                n570 = And(x=w799, y=w805) -> (x .and. y?=w808:bool)
                                n571 = case shown="True" w808 {
                                tunnel: w810 -> [_ w821]
                                frame False {
                                n572 = local write "Temperature Control 5"(FALSE ("Temperature Control 5")) -> ()
                                }
                                frame True {
                                n573 = local write "Temperature SP 5"(w821) -> ()
                                n574 = local write "Temperature Control 5"(TRUE ("Temperature Control 5")) -> ()
                                }
                                }
                                n575 = Wait (ms)(milliseconds to wait=u32 300) -> ()  [unwired: 1 out]
                              }
                            }
                          }
                          frame #1 {
                            # "Wait till Steady State temperature readings on all bays"
                            n576 = while {
                              tunnel: w824 -> [w825]
                              stop <- w826 stop-if-true
                              n577 = flat-sequence {
                                tunnel: [w829] -> w826
                                tunnel: w825 -> [w828]
                                frame #0 {
                                n578 = Wait (ms)(milliseconds to wait=u32 1500) -> ()  [unwired: 1 out]
                                }
                                frame #1 {
                                n579 = local read "Temp SS? 2"() -> (w832:bool)
                                n580 = local read "Temp SS? 3"() -> (w833:bool)
                                n581 = local read "Temp SS? 4"() -> (w834:bool)
                                n582 = local read "Temp SS? 5"() -> (w835:bool)
                                n583 = local read "Temp SS? 1"() -> (w831:bool)
                                n584 = Not(x=w828) -> (.not. x?=w841:bool)
                                n585 = local read "Stop"() -> (w830:bool)
                                n586 = And(x=w833, y=w834) -> (x .and. y?=w837:bool)
                                n587 = And(x=w831, y=w832) -> (x .and. y?=w838:bool)
                                n588 = And(x=w838, y=w837) -> (x .and. y?=w836:bool)
                                n589 = And(x=w836, y=w835) -> (x .and. y?=w839:bool)
                                n590 = Or(x=w841, y=w839) -> (x .or. y?=w840:bool)
                                n591 = Or(x=w840, y=w830) -> (x .or. y?=w829:bool)
                                }
                              }
                            }
                            n592 = local write "Calculate condition"(TRUE ("Calculate condition")) -> ()
                          }
                          frame #2 {
                            n593 = flat-sequence {
                              tunnel: w844 -> [w846]
                              tunnel: [w846] -> w843
                              tunnel: w843 -> [w853]
                              tunnel: [w853] -> w842
                              frame #0 {
                                n594 = local write "Equlibrating Temperature"(TRUE) -> ()
                              }
                              frame #1 {
                                # "Wait 1.5 system volumes"
                                n595 = local read "Number of System Flushes per condtion"() -> (w850:dbl)
                                n596 = local read "Extra system dead volume"() -> (w851:dbl)
                                n597 = script code="start = tic;\nP_tot = P1+P2+P3+P4+P5+P6;\nif P_tot >0\n  extra_res = extr_sys_dead_vol/P_tot;\nelse\n   extra_res =0;\nend\ntotal_sys_res = tau1 + tau2 + tau3 + tau4 + tau5 + extra_res;\ntotal_wait_time = total_sys_res*num_flush_per_cond*60;"("extr_sys_dead_vol"=w851, "num_flush_per_cond"=w850) -> ("??"=w854:errorcluster, "total_wait_time"=w848:dbl, "total_sys_res"=→"Total System Resisdence Time(min)":dbl)  [unwired: 1 in]
                                n598 = Divide(x=w848, y=60.0) -> (x/y=→"total_flush_time":dbl)
                                n599 = while {
                                tunnel: w853 -> [w856]
                                tunnel: w854 -> [w859]
                                stop <- w860 stop-if-true
                                # "Check if system is flushed every 10 seconds"
                                n600 = script code="end1 = toc(start);\nflush_time = 0;\nif end1 > total_wait_time\n   flush_time = 1;\nend\ncurr_wait_time = end1 /60;"("??"=w859) -> ("flush_time"=w863:dbl, "curr_wait_time"=w858:dbl)  [unwired: 1 out]
                                "curr_wait_time" <- w858
                                n601 = Not Equal To 0?(x=w863) -> (x != 0?=w862:bool)
                                n602 = Multiply(x=60.0, y=w858) -> ()  [unwired: 1 out]
                                n603 = local read "Stop"() -> (w865:bool)
                                n604 = Or(x=w862, y=w865) -> (x .or. y?=w861:bool)
                                n605 = Not(x=w856) -> (.not. x?=w855:bool)
                                n606 = Wait (ms)(milliseconds to wait=u32 5000) -> ()  [unwired: 1 out]
                                n607 = Or(x=w861, y=w855) -> (x .or. y?=w860:bool)
                                }
                              }
                            }
                          }
                          frame #3 {
                            n608 = flat-sequence {
                              tunnel: w866 -> [w870]
                              tunnel: w867 -> [w871]
                              tunnel: w866 -> [w880]
                              frame #0 {
                                n609 = script code="start = tic;"() -> ()  [unwired: 1 in, 1 out]
                                n610 = call-poly <vilib>:"PWM Set Duty Cycle.vi"("Duty Cycle (0-1)"=1.0, "PWM Channel"=u8 3, "LINX Resource"=w870) -> ()  [unwired: 7 in, 2 out]
                              }
                              frame #1 {
                                n611 = while {
                                tunnel: w871 -> [w872]
                                stop <- w877 stop-if-true
                                n612 = script code="total_wait_time2 = total_sys_res*1.2*60;\nend1 = toc(start);\nflush_time = 0;\nif end1 > total_wait_time2\n   flush_time = 1;\nend\ncurr_wait_time = end1 /60;"() -> ("flush_time"=w875:dbl)  [unwired: 1 in, 2 out]
                                n613 = Wait (ms)(milliseconds to wait=u32 5000) -> ()  [unwired: 1 out]
                                n614 = local read "Stop"() -> (w876:bool)
                                n615 = Not Equal To 0?(x=w875) -> (x != 0?=w874:bool)
                                n616 = Or(x=w874, y=w876) -> (x .or. y?=w879:bool)
                                n617 = Not(x=w872) -> (.not. x?=w878:bool)
                                n618 = Or(x=w879, y=w878) -> (x .or. y?=w877:bool)
                                }
                              }
                              frame #2 {
                                n619 = call-poly <vilib>:"PWM Set Duty Cycle.vi"("Duty Cycle (0-1)"=0.0, "PWM Channel"=u8 3, "LINX Resource"=w880) -> ()  [unwired: 7 in, 2 out]
                              }
                            }
                          }
                          frame #4 {
                            # "Collect HPLC Data"
                            n620 = flat-sequence {
                              tunnel: w885 -> [w894]
                              tunnel: w884 -> [w893]
                              tunnel: w883 -> [w892]
                              tunnel: w883 -> [w891]
                              frame #0 {
                                n621 = local read "pause for ms"() -> (w888:bool)
                                n622 = case shown="True" w888 {
                                frame False {
                                }
                                frame True {
                                n623 = One Button Dialog(message="Press OK to Analyze Data", button name ("OK")="OK" ("Left Button Text (\"Yes\")")) -> ()  [unwired: 1 out]
                                }
                                }
                                n624 = local write "Flushing System"(TRUE ("Flushing System")) -> ()
                                "System Flushed?" <- TRUE ("System Flushed?")
                              }
                              frame #1 {
                                n625 = flat-sequence {
                                tunnel: w894 -> [w899]
                                tunnel: w893 -> [_]
                                tunnel: w892 -> [w898]
                                tunnel: w891 -> [w897]
                                frame #0 {
                                }
                                frame #1 {
                                n626 = flat-sequence {
                                tunnel: w899 -> [w900]
                                tunnel: w898 -> [w972]
                                tunnel: w899 -> [_]
                                tunnel: [w992] -> w896
                                tunnel: [w991] -> w895
                                tunnel: w897 -> [w990]
                                tunnel: w896 -> [w1025]
                                tunnel: w895 -> [w1024]
                                frame #0 {
                                n627 = local read "COMM Port :: Milligat Pumps"() -> (w902:refnum<visa-resource-name>)
                                n628 = stacked-sequence {
                                tunnel: w902 -> [w905 w917 w935 w940 w949 w962]
                                tunnel: w900 -> [w904 w913 w932 w942 w951 w958]
                                tunnel: 1.0 ("Flowrate(ul/min)") -> [w903 w912 w930 w939 w948 w957]
                                frame #0 {
                                n629 = Index Array(array=w904, index=0) -> (element=w907:dbl)
                                n630 = Greater Than 0?(x=w907) -> (x > 0?=w906:bool)
                                n631 = case shown="True" w906 {
                                tunnel: w905 -> [_ w910]
                                tunnel: w903 -> [_ w909]
                                frame False {
                                }
                                frame True {
                                n632 = call "PumpDispense.vi"("Flowrate(ul/min)"=w909, "Pump Address"="f", "Pump COMM Port"=w910) -> ()  [unwired: 7 in, 2 out]
                                }
                                }
                                }
                                frame #1 {
                                n633 = Index Array(array=w913, index=1) -> (element=w915:dbl)
                                n634 = Greater Than 0?(x=w915) -> (x > 0?=w914:bool)
                                n635 = case shown="True" w914 {
                                tunnel: w912 -> [_ w919]
                                tunnel: w917 -> [_ w918]
                                frame False {
                                }
                                frame True {
                                n636 = local read "Syringe_pump?"() -> (w920:bool)
                                n637 = case shown="False" w920 {
                                tunnel: w919 -> [w921 _]
                                tunnel: w918 -> [w922 _]
                                frame False {
                                n638 = call "PumpDispense.vi"("Flowrate(ul/min)"=w921, "Pump Address"="j", "Pump COMM Port"=w922) -> ()  [unwired: 7 in, 2 out]
                                }
                                frame True {
                                w929 = u16 0 items=["Infuse", "Withdraw"] ("Run Direction (0:Infuse)")
                                w925 = u32 4 items=["milliliters per hour (ml/hr)", "milliliters per minute (ml/min)", "milliliters per second (ml/sec)", "microliters per hour (ul/hr)", "microliters per minute (ul/min)", "microliters per second (ul/sec)", "nanoliters per hour (nl/hr)", "nanoliters per minute (nl/min)", "nanoliters per second (nl/sec)", "picoliters per hour (pl/hr)", "picoliters per minute (pl/min)", "picoliters per second (pl/sec)"] ("Flow Rate Units (1:ml/min)")
                                w926 = u16 0 items=["Infuse", "Withdraw"] ("Pump Direction (0:Infuse)")
                                n639 = local read "COMM Port:: Harvard Syringe Pump"() -> (w927:refnum<visa-resource-name>)
                                n640 = call <instrlib>:"Configure Flow Rate & Direction.vi"("VISA resource name"=w927, "Pump Direction (0:Infuse)"=w926, "Flow Rate (5.00)"=i8 2 ("Pump Address"), "Flow Rate Units (1:ml/min)"=w925) -> ("VISA resource name out"=w928:refnum<visa-resource-name>)  [unwired: 10 in, 1 out]
                                n641 = call <instrlib>:"Start Pump.vi"("Run Direction (0:Infuse)"=w929, "VISA resource name"=w928) -> ()  [unwired: 8 in, 2 out]
                                }
                                }
                                }
                                }
                                }
                                frame #2 {
                                n642 = Index Array(array=w932, index=2) -> (element=w933:dbl)
                                n643 = Greater Than 0?(x=w933) -> (x > 0?=w931:bool)
                                n644 = case shown="True" w931 {
                                tunnel: w935 -> [_ w937]
                                tunnel: w930 -> [_ w936]
                                frame False {
                                }
                                frame True {
                                n645 = call "PumpDispense.vi"("Flowrate(ul/min)"=w936, "Pump Address"="i", "Pump COMM Port"=w937) -> ()  [unwired: 7 in, 2 out]
                                }
                                }
                                }
                                frame #3 {
                                n646 = Index Array(array=w942, index=3) -> (element=w943:dbl)
                                n647 = Greater Than 0?(x=w943) -> (x > 0?=w941:bool)
                                n648 = case shown="False" w941 {
                                tunnel: w940 -> [_ w946]
                                tunnel: w939 -> [_ w945]
                                frame False {
                                }
                                frame True {
                                n649 = call "PumpDispense.vi"("Flowrate(ul/min)"=w945, "Pump Address"="g", "Pump COMM Port"=w946) -> ()  [unwired: 7 in, 2 out]
                                }
                                }
                                }
                                frame #4 {
                                n650 = Index Array(array=w951, index=4) -> (element=w952:dbl)
                                n651 = Greater Than 0?(x=w952) -> (x > 0?=w950:bool)
                                n652 = case shown="True" w950 {
                                tunnel: w949 -> [_ w955]
                                tunnel: w948 -> [_ w954]
                                frame False {
                                }
                                frame True {
                                n653 = call "PumpDispense.vi"("Flowrate(ul/min)"=w954, "Pump Address"="e", "Pump COMM Port"=w955) -> ()  [unwired: 7 in, 2 out]
                                }
                                }
                                }
                                frame #5 {
                                n654 = Index Array(array=w958, index=5) -> (element=w960:dbl)
                                n655 = Greater Than 0?(x=w960) -> (x > 0?=w959:bool)
                                n656 = case shown="True" w959 {
                                tunnel: w962 -> [_ w964]
                                tunnel: w957 -> [_ w963]
                                frame False {
                                }
                                frame True {
                                n657 = call "PumpDispense.vi"("Flowrate(ul/min)"=w963, "Pump Address"="h", "Pump COMM Port"=w964) -> ()  [unwired: 7 in, 2 out]
                                }
                                }
                                }
                                }
                                }
                                frame #1 {
                                n658 = while {
                                stop <- w971 stop-if-true
                                n659 = local read "Phase_Sensor_voltage"() -> (w966:dbl)
                                n660 = script code="organic_phase = 0;\nif start_phase_time \n   start_phase_timer = tic;\n   start_phase_time = 0;\nelse\n  %ignore phase sensor values\n  %if not(phase_sensor_val >2.9 && phase_sensor_val <3.8)\n    %    start_phase_timer = tic;\n   %end\n\n   end_phase_time =  toc(start_phase_timer )\n\n   if end_phase_time > 2\n       organic_phase = 1;\n       start_phase_time = 1;\n   end\n\nend"("phase_sensor_val"=w966) -> ("organic_phase"=w968:dbl)  [unwired: 1 in, 1 out]
                                n661 = local read "Stop"() -> (w970:bool)
                                n662 = Not Equal To 0?(x=w968) -> (x != 0?=w969:bool)
                                n663 = Or(x=w969, y=w970) -> (x .or. y?=w971:bool)
                                n664 = Wait (ms)(milliseconds to wait=u32 300) -> ()  [unwired: 1 out]
                                }
                                }
                                frame #2 {
                                n665 = local read "Stop"() -> (w974:bool)
                                n666 = Not(x=w974) -> (.not. x?=w973:bool)
                                n667 = local read "Sample Valve COMM::Port"() -> (w975:refnum<visa-resource-name>)
                                n668 = case shown="True" w973 {
                                tunnel: w975 -> [_ w977]
                                tunnel: w972 -> [_ w976]
                                frame False {
                                }
                                frame True {
                                n669 = flat-sequence {
                                tunnel: w976 -> [w979]
                                tunnel: w977 -> [w989]
                                frame #0 {
                                n670 = local read "Sample Valve COMM::Port"() -> (w978:refnum<visa-resource-name>)
                                n671 = flat-sequence {
                                tunnel: w981 -> [w986]
                                tunnel: [w986] -> w980
                                frame #0 {
                                n672 = Wait (ms)(milliseconds to wait=u32 500) -> ()  [unwired: 1 out]
                                }
                                }
                                n673 = call-poly <vilib>:"Digital Write.vi"("Output Value"=FALSE, "DO Channel"=u8 22, "LINX Resource"=w980) -> ()  [unwired: 7 in, 2 out]
                                n674 = call-poly <vilib>:"Digital Write.vi"("Output Value"=TRUE, "DO Channel"=u8 22, "LINX Resource"=w979) -> ("LINX Resource"=w981:T10)  [unwired: 7 in, 1 out]
                                n675 = call "NanoValve Inject.vi"("VISA resource name"=w978) -> ()  [unwired: 10 in, 1 out]
                                }
                                frame #1 {
                                n676 = Wait (ms)(milliseconds to wait=u32 2000) -> ()  [unwired: 1 out]
                                }
                                frame #2 {
                                n677 = call "NanoValve Load.vi"("VISA resource name"=w989) -> ()  [unwired: 10 in, 1 out]
                                }
                                }
                                }
                                }
                                }
                                frame #3 {
                                n678 = local read "Stop"() -> (w995:bool)
                                n679 = local read "Bay Parameters"() -> (w991:T2)
                                n680 = Unbundle By Name(w991) -> ("Hplc Wait time(min)"=w993:dbl)
                                n681 = Not(x=w995) -> (.not. x?=w994:bool)
                                n682 = case shown="True" w994 {
                                tunnel: w993 -> [_ w1000]
                                tunnel: [errorcluster {"status"=FALSE, "code"=0, "source"=""} ("error out") w999] -> w992
                                tunnel: w991 -> [_ w998]
                                tunnel: w990 -> [_ w997]
                                frame False {
                                }
                                frame True {
                                n683 = flat-sequence {
                                tunnel: w1000 -> [w1002]
                                tunnel: w997 -> [w1011]
                                tunnel: [w1022] -> w999
                                tunnel: w998 -> [w1021]
                                frame #0 {
                                # "Wait till for HPLC Method"
                                n684 = script code="start = tic;"() -> ("??"=w1001:errorcluster)  [unwired: 1 in]
                                n685 = while {
                                tunnel: w1002 -> [w1004]
                                tunnel: w1001 -> [w1003]
                                stop <- w1010 stop-if-true
                                n686 = Multiply(x=w1004, y=60.0) -> (x*y=w1005:dbl)
                                n687 = script code="end1 = toc(start);\nflush_time = 0;\nif end1 > hplc_wait_time\n   flush_time = 1;\nend"("??"=w1003, "hplc_wait_time"=w1005) -> ("flush_time"=w1007:dbl)  [unwired: 1 out]
                                n688 = local read "Stop"() -> (w1009:bool)
                                n689 = Not Equal To 0?(x=w1007) -> (x != 0?=w1008:bool)
                                n690 = Or(x=w1008, y=w1009) -> (x .or. y?=w1010:bool)
                                }
                                }
                                frame #1 {
                                n691 = flat-sequence {
                                tunnel: w1013 -> [w1018]
                                tunnel: [w1018] -> w1012
                                frame #0 {
                                n692 = Wait (ms)(milliseconds to wait=u32 500) -> ()  [unwired: 1 out]
                                }
                                }
                                n693 = call-poly <vilib>:"Digital Write.vi"("Output Value"=FALSE, "DO Channel"=u8 24, "LINX Resource"=w1011) -> ("LINX Resource"=w1013:T10)  [unwired: 7 in, 1 out]
                                n694 = call-poly <vilib>:"Digital Write.vi"("Output Value"=TRUE, "DO Channel"=u8 24, "LINX Resource"=w1012) -> ()  [unwired: 7 in, 2 out]
                                }
                                frame #2 {
                                n695 = Wait (ms)(milliseconds to wait=u32 30000) -> ()  [unwired: 1 out]
                                }
                                frame #3 {
                                n696 = Unbundle By Name(w1021) -> ("hplc File Name"=w1023:string)
                                n697 = call "hplc_analyze.vi"("File Path"=w1023) -> ("error out"=w1022:errorcluster)  [unwired: 10 in]
                                }
                                }
                                }
                                }
                                }
                                frame #4 {
                                n698 = Unbundle By Name(w1025) -> ("status"=w1026:bool)
                                n699 = case shown="False" w1026 {
                                tunnel: w1024 -> [_ w1027]
                                frame False {
                                }
                                frame True {
                                n700 = while {
                                tunnel: w1027 -> [w1029]
                                stop <- w1028 stop-if-true
                                w1034 = "An error occured while trying to read HPLC data. " ("message")
                                n701 = local write "Error Message"(w1034) -> ()
                                n702 = call <vilib>:"Three Button Dialog.vi"("Right Button Text (\"Cancel\")"="STOP EXPs" ("F button name (\"Cancel\")"), "Center Button Text (\"No\")"="REDO" ("T button name (\"OK\")"), "Left Button Text (\"Yes\")"="REREAD" ("T button name (\"OK\")"), "message"=w1034) -> ("Which Button?"=w1030:T19)  [unwired: 7 in]
                                n703 = case shown="\"Left Button\"" w1030 {
                                tunnel: w1029 -> [_ _ w1041 _]
                                tunnel: [TRUE TRUE w1040 w1043] -> w1028
                                frame "Right Button" {
                                w1035 = TRUE ("Setup Error")
                                n704 = local write "System Error"(w1035) -> ()
                                n705 = local write "Setup Error"(w1035) -> ()
                                n706 = script code="system_error = 1"() -> ()  [unwired: 1 in, 1 out]
                                n707 = local write "Stop"(w1035) -> ()
                                }
                                frame "Center Button" {
                                n708 = script code="redo = true;\nopt_ctr = 1;\nCurrExp = CurrExp + 1;\nncall0 = ncall0 +1;\nif req_ctr == req_tot\n       opt_ctr = 3;\n  else\n     req_ctr = req_ctr +1;\nend"() -> ()  [unwired: 1 in, 1 out]
                                }
                                frame "Left Button" {
                                n709 = Unbundle By Name(w1041) -> ("hplc File Name"=w1042:string)
                                n710 = call "hplc_analyze.vi"("File Path"=w1042) -> ("error out"=w1038:errorcluster)  [unwired: 10 in]
                                n711 = Unbundle By Name(w1038) -> ("status"=w1039:bool)
                                n712 = Not(x=w1039) -> (.not. x?=w1040:bool)
                                }
                                frame "Window Close" {
                                w1043 = TRUE
                                n713 = local write "Setup Error"(w1043) -> ()
                                n714 = script code="system_error = 1"() -> ()  [unwired: 1 in, 1 out]
                                n715 = local write "Stop"(w1043) -> ()
                                }
                                }
                                }
                                }
                                }
                                }
                                frame #5 {
                                n716 = disable-structure shown="Disabled" {
                                frame Disabled {
                                n717 = flat-sequence {
                                tunnel: w1045 -> [w1050]
                                tunnel: [w1050] -> w1044
                                frame #0 {
                                n718 = Wait (ms)(milliseconds to wait=u32 500) -> ()  [unwired: 1 out]
                                }
                                }
                                n719 = call-poly <vilib>:"Digital Write.vi"("Output Value"=FALSE, "DO Channel"=u8 22) -> ("LINX Resource"=w1045:T10)  [unwired: 8 in, 1 out]
                                n720 = call-poly <vilib>:"Digital Write.vi"("Output Value"=TRUE, "DO Channel"=u8 22, "LINX Resource"=w1044) -> ()  [unwired: 7 in, 2 out]
                                }
                                frame Enabled {
                                }
                                }
                                }
                                }
                                }
                                }
                              }
                              frame #2 {
                                n721 = local read "Stop"() -> (w1053:bool)
                                n722 = local write "HPLC Analysis"(TRUE ("HPLC Analysis")) -> ()
                                n723 = Not(x=w1053) -> (.not. x?=w1052:bool)
                                n724 = case shown="True" w1052 {
                                frame False {
                                }
                                frame True {
                                n725 = script code="C_measured =Conc;\nFvalues(end +1,:) = [Conc];"() -> ()  [unwired: 1 in, 1 out]
                                }
                                }
                              }
                            }
                          }
                          frame #5 {
                            n726 = local read "Stop"() -> (w1056:bool)
                            n727 = Not(x=w1056) -> (.not. x?=w1055:bool)
                            n728 = case shown="True" w1055 {
                              tunnel: [1.0 w1067] -> w1057
                              frame False {
                              }
                              frame True {
                                # "Save data to excel file"
                                n729 = local read "Bay Parameters"() -> (w1065:T2)
                                n730 = Unbundle By Name(w1065) -> ("Total Number of Experiments 2"=w1064:dbl)
                                n731 = script code="analyze_labview_results"("ncall"=w1064) -> ("terminate"=w1067:dbl, "ncall0"=w1066:dbl, "experiment_history"=w1062:dbl[][], "Pbest"=w1060:dbl[], "Tbest"=w1061:dbl[], "best_exp_num"=w1059:dbl)  [unwired: 1 in, 1 out]
                                n732 = local write "Flowrates(ul/min)_best"(w1060) -> ()
                                n733 = local write "temperature_best"(w1061) -> ()
                                n734 = local write "best_exp_num"(w1059) -> ()
                                n735 = local write "Current Experiment"(w1066) -> ()
                                n736 = local write "Total Number of Experiments"(w1064) -> ()
                                n737 = call-poly <vilib>:"Array To Matrix.vi"("Real 2D Array"=w1062) -> ("Real Matrix"=w1063:T18)
                                n738 = local write "experiment history"(w1063) -> ()
                              }
                            }
                          }
                          frame #6 {
                            n739 = local read "Num_exp_till_pause"() -> (w1069:i32)
                            n740 = Increment(x=w1069) -> (x+1=w1068:i32)
                            n741 = local write "Num_exp_till_pause"(w1068) -> ()
                          }
                          frame #7 {
                            # "Pause System"
                            n742 = local read "Bay Parameters"() -> (w1077:T2)
                            n743 = Unbundle By Name(w1077) -> ("Num_conditons_per_wait"=w1076:dbl)
                            n744 = local read "Num_exp_till_pause"() -> (w1075:i32)
                            n745 = Equal?(x=w1076, y=w1075) -> (x = y?=w1074:bool)
                            n746 = local read "Run_Stop_cluster"() -> (w1071:T7)
                            n747 = Unbundle By Name(w1071) -> ("Stop Run Button"=w1073:bool)
                            n748 = Or(x=w1073, y=w1074) -> (x .or. y?=w1072:bool)
                            n749 = case shown="True" w1072 {
                              tunnel: w1076 -> [w1080 _]
                              tunnel: w1075 -> [w1081 _]
                              tunnel: w1071 -> [_ w1083]
                              frame False {
                                n750 = Greater?(x=w1081, y=w1080) -> (0:w1079:bool)
                                n751 = case shown="True" w1079 {
                                frame False {
                                }
                                frame True {
                                n752 = local write "Num_exp_till_pause"(0 ("Num_exp_till_pause")) -> ()
                                }
                                }
                              }
                              frame True {
                                n753 = flat-sequence {
                                tunnel: w1083 -> [w1111]
                                frame #0 {
                                w1087 = string[] ["e", "f", "g", "h", "i", "j"]
                                # "Turn off pumps and stop controling temperature"
                                n754 = stacked-sequence {
                                frame #0 {
                                n755 = local write "Temperature Control 1"(FALSE ("Temperature Control 1")) -> ()
                                }
                                frame #1 {
                                n756 = local write "Temperature Control 2"(FALSE ("Temperature Control 2")) -> ()
                                }
                                frame #2 {
                                n757 = local write "Temperature Control 3"(FALSE ("Temperature Control 3")) -> ()
                                }
                                frame #3 {
                                n758 = local write "Temperature Control 4"(FALSE ("Temperature Control 4")) -> ()
                                }
                                frame #4 {
                                n759 = local write "Temperature Control 5"(FALSE ("Temperature Control 5")) -> ()
                                }
                                }
                                n760 = local read "COMM Port:: Harvard Syringe Pump"() -> (w1085:refnum<visa-resource-name>)
                                n761 = local read "Syringe_pump?"() -> (w1084:bool)
                                n762 = local read "COMM Port :: Milligat Pumps"() -> (w1086:refnum<visa-resource-name>)
                                n763 = Array Size(array=w1087) -> (size(s)=w1088:i32)
                                n764 = case shown="True" w1084 {
                                tunnel: w1085 -> [_ w1096]
                                frame False {
                                }
                                frame True {
                                n765 = call <instrlib>:"Stop Pump.vi"("VISA resource name"=w1096) -> ()  [unwired: 9 in, 2 out]
                                }
                                }
                                n766 = for {
                                N: w1088 -> [_]
                                tunnel: w1087 -> [w1094] mode=indexing
                                tunnel: w1086 -> [w1095]
                                n767 = call "PumpStop.vi"("Pump Address"=w1094, "Pump COMM Port"=w1095) -> ()  [unwired: 9 in, 1 out]
                                }
                                }
                                frame #1 {
                                n768 = local read "Stop"() -> (w1099:bool)
                                n769 = Not(x=w1099) -> (.not. x?=w1098:bool)
                                n770 = case shown="True" w1098 {
                                frame False {
                                }
                                frame True {
                                n771 = while {
                                stop <- w1105 stop-if-true
                                # "Wait till user confirms system resume"
                                n772 = Two Button Dialog(message="System is currently paused. Refill Syringes, flush lines, then press OK to continue optimization.\nOr Redo to repeat condition ", 1:"REDO" ("F button name (\"Cancel\")"), 2:"OK" ("Left Button Text (\"Yes\")")) -> (T button?=w1101:bool)
                                n773 = case shown="False" w1101 {
                                tunnel: [TRUE TRUE] -> w1100
                                frame False {
                                n774 = script code="redo = true;"() -> ()  [unwired: 1 in, 1 out]
                                }
                                frame True {
                                }
                                }
                                n775 = local read "Stop"() -> (w1106:bool)
                                n776 = Or(x=w1100, y=w1106) -> (x .or. y?=w1105:bool)
                                }
                                }
                                }
                                n777 = local write "stop_xl_write"(TRUE ("stop_xl_write")) -> ()
                                }
                                frame #2 {
                                n778 = local write "Num_exp_till_pause"(0 ("Num_exp_till_pause")) -> ()
                                n779 = Bundle By Name(cluster=w1111, "Stop Run Button"=FALSE) -> (w1109:T7)
                                n780 = local write "Run_Stop_cluster"(w1109) -> ()
                                }
                                }
                              }
                            }
                          }
                          frame #8 {
                            w1114 = FALSE
                            n781 = local write "Equlibrating Temperature"(w1114) -> ()
                            n782 = local write "Calculate condition"(w1114) -> ()
                            n783 = local write "Flushing System"(w1114) -> ()
                            n784 = local write "HPLC Analysis"(w1114) -> ()
                            n785 = local write "stop_xl_write"(TRUE ("stop_xl_write")) -> ()
                          }
                        }
                        n786 = while {
                          stop <- w1141 stop-if-true
                          n787 = flat-sequence {
                            frame #0 {
                              n788 = script code="save_excel_time_data;"() -> ()  [unwired: 1 in, 1 out]
                            }
                            frame #1 {
                              n789 = Wait (ms)(milliseconds to wait=u32 30000) -> ()  [unwired: 1 out]
                            }
                          }
                          n790 = local read "Stop"() -> (w1142:bool)
                          n791 = local read "stop_xl_write"() -> (w1140:bool)
                          n792 = Or(x=w1140, y=w1142) -> (x .or. y?=w1141:bool)
                        }
                      }
                    }
                  }
                }
                n793 = Greater?(x=w609, y=w610) -> (0:w617:bool)
                n794 = Equal?(x=w615, y=1.0) -> (x = y?=w611:bool)
                n795 = local read "Stop"() -> (w618:bool)
                n796 = Or(x=w618, y=w617) -> (x .or. y?=w614:bool)
                n797 = Or(x=w611, y=w614) -> (x .or. y?=w613:bool)
                n798 = case shown="True" w611 {
                  frame False {
                  }
                  frame True {
                    w622 = u16 2 items=["System  Error", "System Running", "System Standby"] ("System Status")
                    n799 = local write "Stop"(TRUE ("Stop")) -> ()
                    n800 = local write "System Status"(w622) -> ()
                  }
                }
                "Optimization_loop_index" <- w619
              }
            }
          }
          n801 = while {
            tunnel: w597 -> [w1237]
            stop <- w1240 stop-if-true
            n802 = local read "Temperature Control 3"() -> (w1238:bool)
            n803 = local read "running?"() -> (w1236:bool)
            n804 = And(x=w1236, y=w1238) -> (x .and. y?=w1239:bool)
            n805 = case shown="True" w1239 {
              tunnel: w1237 -> [_ w1243]
              frame False {
                n806 = local write "Temp SS? 3"(TRUE) -> ()
              }
              frame True {
                # "Bay 3 Temperature Controller"
                n807 = local read "Temperature SP 3"() -> (w1244:dbl)
                n808 = local read "Temperature 3"() -> (w1247:dbl)
                n809 = Subtract(x=w1247, y=w1244) -> (x-y=w1256:dbl)
                n810 = Absolute Value(x=w1256) -> (abs(x)=w1258:dbl)
                n811 = Less Or Equal?(x=w1258, y=1.2) -> (x <= y?=w1255:bool)
                n812 = local write "Temp SS? 3"(w1255) -> ()
                n813 = local read "SSR Duration 3"() -> (w1265:dbl)
                n814 = call-poly <vilib>:"PID Online Autotuning.vi"("setpoint"=w1244, "manipulated variable"=w1265, "autotuning parameters"=T9 {"type of controller"=enum."PID", "relay cycles"=3, "relay amplitude"=1.0, "control specifications"=enum."Normal", "PV noise level"=0.1} ("Autotuning Parameters R1"), "process variable"=w1247, "PID gains in"=T8 {"Proportional gain Kc"=0.38538, "Integral time Ti (sec)"=0.524375, "Derivative time Ti (sec)"=0.12585} ("PID gains 2")) -> ("setpoint out"=w1263:dbl, "process variable out"=w1264:dbl, "PID gains out"=w1267:T17)  [unwired: 6 in, 2 out]
                n815 = Greater?(x=w1244, y=w1247) -> (0:w1254:bool)
                n816 = call <vilib>:"PID Autotuning (Temperature).vi"("desired temperature"=w1263, "measured temperature"=w1264, "PID gains in"=w1267, "output range"=cluster{"output high":dbl, "output low":dbl} {"output high"=3.0, "output low"=-1.0} ("Output range")) -> ("output"=w1260:dbl)  [unwired: 12 in, 3 out]
                n817 = Multiply(x=1000.0, y=w1260) -> (x*y=w1262:dbl)
                n818 = local write "SSR Duration 3"(w1260) -> ()
                n819 = Greater Than 0?(x=w1262) -> (x > 0?=w1253:bool)
                n820 = And(x=w1253, y=w1254) -> (x .and. y?=w1251:bool)
                n821 = Subtract(x=w1247, y=10.0) -> (x-y=w1249:dbl)
                n822 = Less?(x=w1249, y=w1244) -> (x < y?=w1252:bool)
                n823 = And(x=w1252, y=w1251) -> (x .and. y?=w1250:bool)
                n824 = case shown="True" w1250 {
                  tunnel: [errorcluster {"status"=FALSE, "code"=0, "source"=""} ("error out") w1279] -> _
                  tunnel: 4 -> [_ w1277]
                  tunnel: w1262 -> [w1273 w1278]
                  tunnel: [0.0 w1281] -> w1245
                  tunnel: w1244 -> [_ w1280]
                  tunnel: w1243 -> [_ w1276]
                  frame False {
                    n825 = Absolute Value(x=w1273) -> (abs(x)=w1274:dbl)
                    n826 = Wait (ms)(milliseconds to wait=w1274) -> ()  [unwired: 1 out]
                  }
                  frame True {
                    n827 = call "TurnOnRelayArduino.vi"("channel"=w1277, "duration"=w1278, "LINX Resource"=w1276) -> ("error out"=w1279:errorcluster)  [unwired: 7 in, 1 out]
                    n828 = script code="tempdiff3= SP3 - T3;\nif tempdiff3 > 10\n  if slope3 < .01\n     temp_check3 = temp_check3 + 1;\n  else\n      temp_check3 =0;\n  end\nend\n\nif temp_check3 > 9\n  temp_error3 = 1\nend"("SP3"=w1280) -> ("temp_error3"=w1281:dbl)  [unwired: 1 in, 1 out]
                  }
                }
                n829 = Not Equal To 0?(x=w1245) -> (x != 0?=w1246:bool)
                n830 = case shown="True" w1246 {
                  frame False {
                  }
                  frame True {
                    n831 = local write "Error Message"("Bay 3 Temperature Heating Error") -> ()
                  }
                }
                n832 = case shown="True" w1246 {
                  tunnel: w1246 -> [_ w1271]
                  frame False {
                  }
                  frame True {
                    n833 = local write "System Error"(w1271) -> ()
                    n834 = local write "Stop"(w1271) -> ()
                  }
                }
              }
            }
            n835 = Wait (ms)(milliseconds to wait=u32 400) -> ()  [unwired: 1 out]
            n836 = local read "Stop"() -> (w1240:bool)
          }
          n837 = while {
            tunnel: w597 -> [w1191]
            stop <- w1194 stop-if-true
            n838 = local read "running?"() -> (w1190:bool)
            n839 = Wait (ms)(milliseconds to wait=u32 400) -> ()  [unwired: 1 out]
            n840 = local read "Temperature Control 4"() -> (w1193:bool)
            n841 = And(x=w1190, y=w1193) -> (x .and. y?=w1192:bool)
            n842 = case shown="True" w1192 {
              tunnel: w1191 -> [_ w1197]
              frame False {
                n843 = local write "Temp SS? 4"(TRUE ("Temp SS? 4")) -> ()
              }
              frame True {
                # "Bay 4 Temperature Controller"
                n844 = local read "Temperature SP 4"() -> (w1200:dbl)
                n845 = local read "Temperature 4"() -> (w1203:dbl)
                n846 = Subtract(x=w1203, y=w1200) -> (x-y=w1210:dbl)
                n847 = Absolute Value(x=w1210) -> (abs(x)=w1212:dbl)
                n848 = Less Or Equal?(x=w1212, y=1.2) -> (x <= y?=w1209:bool)
                n849 = local write "Temp SS? 4"(w1209) -> ()
                n850 = local read "SSR Duration 4"() -> (w1213:dbl)
                n851 = call-poly <vilib>:"PID Online Autotuning.vi"("setpoint"=w1200, "manipulated variable"=w1213, "autotuning parameters"=T9 {"type of controller"=enum."PID", "relay cycles"=3, "relay amplitude"=1.0, "control specifications"=enum."Normal", "PV noise level"=0.1} ("Autotuning Parameters R1"), "process variable"=w1203, "PID gains in"=T8 {"Proportional gain Kc"=0.38538, "Integral time Ti (sec)"=0.524375, "Derivative time Ti (sec)"=0.12585} ("PID gains 2")) -> ("setpoint out"=w1215:dbl, "process variable out"=w1216:dbl, "PID gains out"=w1218:T17)  [unwired: 6 in, 2 out]
                n852 = call <vilib>:"PID Autotuning (Temperature).vi"("desired temperature"=w1215, "measured temperature"=w1216, "PID gains in"=w1218, "output range"=cluster{"output high":dbl, "output low":dbl} {"output high"=3.0, "output low"=-1.0} ("Output range")) -> ("output"=w1214:dbl)  [unwired: 12 in, 3 out]
                n853 = Subtract(x=w1203, y=10.0) -> (x-y=w1202:dbl)
                n854 = Less?(x=w1202, y=w1200) -> (x < y?=w1204:bool)
                n855 = Multiply(x=1000.0, y=w1214) -> (x*y=w1222:dbl)
                n856 = Greater?(x=w1200, y=w1203) -> (0:w1208:bool)
                n857 = Greater Than 0?(x=w1222) -> (x > 0?=w1207:bool)
                n858 = local write "SSR Duration 4"(w1214) -> ()
                n859 = And(x=w1207, y=w1208) -> (x .and. y?=w1206:bool)
                n860 = And(x=w1204, y=w1206) -> (x .and. y?=w1205:bool)
                n861 = case shown="True" w1205 {
                  tunnel: [errorcluster {"status"=FALSE, "code"=0, "source"=""} ("error out") w1233] -> _
                  tunnel: 5 -> [_ w1231]
                  tunnel: w1222 -> [w1227 w1232]
                  tunnel: w1200 -> [_ w1235]
                  tunnel: [0.0 w1234] -> w1199
                  tunnel: w1197 -> [_ w1230]
                  frame False {
                    n862 = Absolute Value(x=w1227) -> (abs(x)=w1228:dbl)
                    n863 = Wait (ms)(milliseconds to wait=w1228) -> ()  [unwired: 1 out]
                  }
                  frame True {
                    n864 = call "TurnOnRelayArduino.vi"("channel"=w1231, "duration"=w1232, "LINX Resource"=w1230) -> ("error out"=w1233:errorcluster)  [unwired: 7 in, 1 out]
                    n865 = script code="tempdiff4= SP4 - T4;\nif tempdiff4 > 10\n  if slope4 < .01\n     temp_check4 = temp_check4 + 1;\n  else\n      temp_check4 =0;\n  end\nend\n\nif temp_check4 > 9\n  temp_error4 = 1\nend"("SP4"=w1235) -> ("temp_error4"=w1234:dbl)  [unwired: 1 in, 1 out]
                  }
                }
                n866 = Not Equal To 0?(x=w1199) -> (x != 0?=w1198:bool)
                n867 = case shown="True" w1198 {
                  frame False {
                  }
                  frame True {
                    n868 = local write "Error Message"("Bay 4 Temperature Heating Error") -> ()
                  }
                }
                n869 = case shown="True" w1198 {
                  tunnel: w1198 -> [_ w1225]
                  frame False {
                  }
                  frame True {
                    n870 = local write "System Error"(w1225) -> ()
                    n871 = local write "Stop"(w1225) -> ()
                  }
                }
              }
            }
            n872 = local read "Stop"() -> (w1194:bool)
          }
          n873 = while {
            stop <- w602 stop-if-true
            n874 = script code="TempArr1=circshift(TempArr1,9);\nTempArr2=circshift(TempArr2,9);\nTempArr3=circshift(TempArr3,9);\nTempArr4=circshift(TempArr4,9);\nTempArr5=circshift(TempArr5,9);\n\nTempArr1(10)=T1;\nTempArr2(10)=T2;\nTempArr3(10)=T3;\nTempArr4(10)=T4;\nTempArr5(10)=T5;\n\n[slope1 temp] = polyfit([1,2,3,4,5,6,7,8,9,10]',TempArr1,1);\nslope1 = slope1(1);\n[slope2 temp] = polyfit([1,2,3,4,5,6,7,8,9,10]',TempArr2,1);\nslope2= slope2(1);\n[slope3 temp] = polyfit([1,2,3,4,5,6,7,8,9,10]',TempArr3,1);\nslope3 = slope3(1);\n[slope4 temp] = polyfit([1,2,3,4,5,6,7,8,9,10]',TempArr4,1);\nslope4 = slope4(1);\n[slope5 temp] = polyfit([1,2,3,4,5,6,7,8,9,10]',TempArr5,1);\nslope5 = slope5(1);"() -> ()  [unwired: 1 in, 1 out]
            n875 = Wait (ms)(milliseconds to wait=u32 600) -> ()  [unwired: 1 out]
            n876 = local read "Stop"() -> (w602:bool)
          }
          n877 = while {
            tunnel: w597 -> [w1145]
            stop <- w1148 stop-if-true
            n878 = local read "running?"() -> (w1144:bool)
            n879 = local read "Temperature Control 5"() -> (w1146:bool)
            n880 = And(x=w1144, y=w1146) -> (x .and. y?=w1147:bool)
            n881 = case shown="True" w1147 {
              tunnel: w1145 -> [_ w1151]
              frame False {
                n882 = local write "Temp SS? 5"(TRUE ("Temp SS? 5")) -> ()
              }
              frame True {
                # "Bay 5 Temperature Controller"
                n883 = local read "SSR Duration 5"() -> (w1167:dbl)
                n884 = local read "Temperature SP 5"() -> (w1153:dbl)
                n885 = local read "Temperature 5"() -> (w1156:dbl)
                n886 = Subtract(x=w1156, y=w1153) -> (x-y=w1164:dbl)
                n887 = Absolute Value(x=w1164) -> (abs(x)=w1166:dbl)
                n888 = Less Or Equal?(x=w1166, y=1.2) -> (x <= y?=w1163:bool)
                n889 = local write "Temp SS? 5"(w1163) -> ()
                n890 = call-poly <vilib>:"PID Online Autotuning.vi"("setpoint"=w1153, "manipulated variable"=w1167, "autotuning parameters"=T9 {"type of controller"=enum."PID", "relay cycles"=3, "relay amplitude"=1.0, "control specifications"=enum."Normal", "PV noise level"=0.1} ("Autotuning Parameters R1"), "process variable"=w1156, "PID gains in"=T8 {"Proportional gain Kc"=0.38538, "Integral time Ti (sec)"=0.524375, "Derivative time Ti (sec)"=0.12585} ("PID gains 2")) -> ("setpoint out"=w1169:dbl, "process variable out"=w1170:dbl, "PID gains out"=w1172:T17)  [unwired: 6 in, 2 out]
                n891 = call <vilib>:"PID Autotuning (Temperature).vi"("desired temperature"=w1169, "measured temperature"=w1170, "PID gains in"=w1172, "output range"=cluster{"output high":dbl, "output low":dbl} {"output high"=3.0, "output low"=-1.0} ("Output range")) -> ("output"=w1168:dbl)  [unwired: 12 in, 3 out]
                n892 = Multiply(x=1000.0, y=w1168) -> (x*y=w1176:dbl)
                n893 = Greater?(x=w1153, y=w1156) -> (0:w1161:bool)
                n894 = Greater Than 0?(x=w1176) -> (x > 0?=w1162:bool)
                n895 = local write "SSR Duration 5"(w1168) -> ()
                n896 = And(x=w1162, y=w1161) -> (x .and. y?=w1159:bool)
                n897 = Subtract(x=w1156, y=10.0) -> (x-y=w1157:dbl)
                n898 = Greater?(x=w1157, y=w1153) -> (0:w1160:bool)
                n899 = And(x=w1160, y=w1159) -> (x .and. y?=w1158:bool)
                n900 = case shown="True" w1158 {
                  tunnel: [errorcluster {"status"=FALSE, "code"=0, "source"=""} ("error out") w1187] -> _
                  tunnel: 6 -> [_ w1184]
                  tunnel: w1176 -> [w1181 w1185]
                  tunnel: [0.0 w1189] -> w1154
                  tunnel: w1153 -> [_ w1188]
                  tunnel: w1151 -> [_ w1186]
                  frame False {
                    n901 = Absolute Value(x=w1181) -> (abs(x)=w1182:dbl)
                    n902 = Wait (ms)(milliseconds to wait=w1182) -> ()  [unwired: 1 out]
                  }
                  frame True {
                    n903 = call "TurnOnRelayArduino.vi"("channel"=w1184, "duration"=w1185, "LINX Resource"=w1186) -> ("error out"=w1187:errorcluster)  [unwired: 7 in, 1 out]
                    n904 = script code="tempdiff5= SP5 - T5;\n\nif tempdiff5 > 10\n  if slope5 < .01\n     temp_check5 = temp_check5 + 1;\n  else\n      temp_check5 =0;\n  end\nend\n\nif temp_check5 >9\n  temp_error5 = 1\nend"("SP5"=w1188) -> ("temp_error5"=w1189:dbl)  [unwired: 1 in, 1 out]
                  }
                }
                n905 = Not Equal To 0?(x=w1154) -> (x != 0?=w1152:bool)
                n906 = case shown="True" w1152 {
                  frame False {
                  }
                  frame True {
                    n907 = local write "Error Message"("Bay 5 Temperature Heating Error") -> ()
                  }
                }
                n908 = case shown="True" w1152 {
                  tunnel: w1152 -> [_ w1179]
                  frame False {
                  }
                  frame True {
                    n909 = local write "Stop"(w1179) -> ()
                    n910 = local write "System Error"(w1179) -> ()
                  }
                }
              }
            }
            n911 = Wait (ms)(milliseconds to wait=u32 400) -> ()  [unwired: 1 out]
            n912 = local read "Stop"() -> (w1148:bool)
          }
        }
      }
      n913 = local read "IR Sensor Device"() -> (w62:T6)
      n914 = while {
        tunnel: errorcluster {"status"=FALSE, "code"=0, "source"=""} ("error out") -> [w140]
        tunnel: w62 -> [w159]
        stop <- w180 stop-if-true
        w137 = u8 7 items=["RAM IR raw  Ch1"=4, "RAM IR raw  Ch2"=5, "RAM T_A"=6, "RAM T_OBJ1"=7, "RAM T_OBJ2"=8, "EEPROM_To_max"=32, "EEPROM_To_min"=33, "EEPROM_PWM_CTRL"=34, "EEPROM_Ta_range"=35, "EEPROM_Emissivity_CorrCoeff"=36, "EEPROM_SMBus Address"=46, "EEPROM_ConfigReg"=37] ("Melexis_Cmmds")
        # "Bay 5 Temperature Read"
        # "Bay 4 Temperature Read"
        # "Bay 3 Temperature Read"
        # "Bay 2 Temperature Read"
        # "Bay 1 Temperature Read"
        n915 = local read "Stop"() -> (w180:bool)
        n916 = call "IRSensorNIRead.vi"("error in (no error)"=w140, "Melexis_Cmmds"=w137, "Address"=u8 1, "device reference"=w159) -> ("error out"=w162:errorcluster, "Temperature"=w160:dbl, "device reference out"=w158:T6)  [unwired: 5 in]
        n917 = local write "error out"(w162) -> ()
        n918 = Unbundle By Name(w162) -> ("status"=w161:bool)
        n919 = call-poly <vilib>:"PID Control Input Filter.vi"("input"=w160) -> ("output"=w173:dbl)  [unwired: 4 in]
        n920 = case shown="False" w161 {
          tunnel: w172 -> [w189 _]
          tunnel: [w189 w190] -> w177
          frame False {
            n921 = local write "Temperature 1"(w189) -> ()
          }
          frame True {
            n922 = local read "Temperature 1"() -> (w190:dbl)
          }
        }
        n923 = flat-sequence {
          tunnel: w173 -> [w203]
          tunnel: [w203] -> w172
          tunnel: w158 -> [w202]
          tunnel: [w202] -> w157
          frame #0 {
            n924 = Wait (ms)(milliseconds to wait=u32 100) -> ()  [unwired: 1 out]
          }
        }
        n925 = call "IRSensorNIRead.vi"("error in (no error)"=w140, "Melexis_Cmmds"=w137, "Address"=u8 2, "device reference"=w157) -> ("error out"=w149:errorcluster, "Temperature"=w150:dbl, "device reference out"=w152:T6)  [unwired: 5 in]
        n926 = local write "error out"(w149) -> ()
        n927 = Unbundle By Name(w149) -> ("status"=w154:bool)
        n928 = call-poly <vilib>:"PID Control Input Filter.vi"("input"=w150) -> ("output"=w171:dbl)  [unwired: 4 in]
        n929 = case shown="True" w154 {
          tunnel: w170 -> [w187 _]
          tunnel: [w187 w188] -> w176
          frame False {
            n930 = local write "Temperature 2"(w187) -> ()
          }
          frame True {
            n931 = local read "Temperature 2"() -> (w188:dbl)
          }
        }
        n932 = flat-sequence {
          tunnel: w171 -> [w200]
          tunnel: [w200] -> w170
          tunnel: w152 -> [w199]
          tunnel: [w199] -> w151
          frame #0 {
            n933 = Wait (ms)(milliseconds to wait=u32 100) -> ()  [unwired: 1 out]
          }
        }
        n934 = call "IRSensorNIRead.vi"("error in (no error)"=w140, "Melexis_Cmmds"=w137, "Address"=u8 3, "device reference"=w151) -> ("error out"=w142:errorcluster, "Temperature"=w148:dbl, "device reference out"=w147:T6)  [unwired: 5 in]
        n935 = local write "error out"(w142) -> ()
        n936 = Unbundle By Name(w142) -> ("status"=w143:bool)
        n937 = case shown="False" w143 {
          tunnel: w167 -> [w185 _]
          tunnel: [w185 w186] -> w169
          frame False {
            n938 = local write "Temperature 3"(w185) -> ()
          }
          frame True {
            n939 = local read "Temperature 3"() -> (w186:dbl)
          }
        }
        n940 = call-poly <vilib>:"PID Control Input Filter.vi"("input"=w148) -> ("output"=w168:dbl)  [unwired: 4 in]
        n941 = flat-sequence {
          tunnel: w168 -> [w197]
          tunnel: [w197] -> w167
          tunnel: w147 -> [w196]
          tunnel: [w196] -> w145
          frame #0 {
            n942 = Wait (ms)(milliseconds to wait=u32 100) -> ()  [unwired: 1 out]
          }
        }
        n943 = call "IRSensorNIRead.vi"("error in (no error)"=w140, "Melexis_Cmmds"=w137, "Address"=u8 4, "device reference"=w145) -> ("error out"=w132:errorcluster, "Temperature"=w144:dbl, "device reference out"=w139:T6)  [unwired: 5 in]
        n944 = local write "error out"(w132) -> ()
        n945 = Unbundle By Name(w132) -> ("status"=w134:bool)
        n946 = case shown="True" w134 {
          tunnel: w165 -> [w183 _]
          tunnel: [w183 w184] -> w175
          frame False {
            n947 = local write "Temperature 4"(w183) -> ()
          }
          frame True {
            n948 = local read "Temperature 4"() -> (w184:dbl)
          }
        }
        n949 = call-poly <vilib>:"PID Control Input Filter.vi"("input"=w144) -> ("output"=w166:dbl)  [unwired: 4 in]
        n950 = flat-sequence {
          tunnel: w166 -> [w194]
          tunnel: [w194] -> w165
          tunnel: w139 -> [w193]
          tunnel: [w193] -> w138
          frame #0 {
            n951 = Wait (ms)(milliseconds to wait=u32 100) -> ()  [unwired: 1 out]
          }
        }
        n952 = call "IRSensorNIRead.vi"("error in (no error)"=w140, "Melexis_Cmmds"=w137, "Address"=u8 5, "device reference"=w138) -> ("error out"=w135:errorcluster, "Temperature"=w136:dbl)  [unwired: 5 in, 1 out]
        n953 = local write "error out"(w135) -> ()
        n954 = flat-sequence {
          tunnel: w164 -> [w191]
          tunnel: [w191] -> w163
          frame #0 {
            n955 = Wait (ms)(milliseconds to wait=u32 100) -> ()  [unwired: 1 out]
          }
        }
        n956 = Unbundle By Name(w135) -> ("status"=w133:bool)
        n957 = call-poly <vilib>:"PID Control Input Filter.vi"("input"=w136) -> ("output"=w164:dbl)  [unwired: 4 in]
        n958 = local write "error out"(w140) -> ()
        n959 = Build Array(w177, w176, w169, w175, w163) -> (w179:dbl[])
        n960 = Array To Cluster(array=w179) -> (cluster=→"Teperature Chart":T3)
        n961 = case shown="False" w133 {
          tunnel: w163 -> [w181 _]
          tunnel: [w181 w182] -> w174
          frame False {
            n962 = local write "Temperature 5"(w181) -> ()
          }
          frame True {
            n963 = local read "Temperature 5"() -> (w182:dbl)
          }
        }
        n964 = script code="MATLAB script"("T1"=w177, "T2"=w176, "T3"=w169, "T4"=w175, "T5"=w174) -> ()  [unwired: 1 in, 1 out]
      }
      n965 = while {
        stop <- w95 stop-if-true
        n966 = local read "Pump setpoint(ul/min) 1"() -> (w98:dbl)
        n967 = local read "Pump setpoint(ul/min) 2"() -> (w94:dbl)
        n968 = local read "Pump setpoint(ul/min) 3"() -> (w93:dbl)
        n969 = local read "Pump setpoint(ul/min) 4"() -> (w92:dbl)
        n970 = local read "Pump setpoint(ul/min) 5"() -> (w91:dbl)
        n971 = local read "Pump setpoint(ul/min) 6"() -> (w90:dbl)
        n972 = Build Array(w98, w94, w93, w92, w91, w90) -> (w99:dbl[])
        n973 = Array To Cluster(array=w99) -> (cluster=→"Pump Setpoints Chart":T3)
        n974 = Wait (ms)(milliseconds to wait=u32 5000) -> ()  [unwired: 1 out]
        n975 = local read "Stop"() -> (w95:bool)
      }
      n976 = while {
        stop <- w77 stop-if-true
        n977 = local read "System Error"() -> (w76:bool)
        n978 = Wait (ms)(milliseconds to wait=u32 300) -> ()  [unwired: 1 out]
        n979 = case shown="True" w76 {
          tunnel: [w81 w82] -> w74
          frame False {
            w78 = u16 2 items=["System  Error", "System Running", "System Standby"] ("System Status")
            w79 = u16 1 items=["System  Error", "System Running", "System Standby"] ("System Status")
            n980 = local read "running?"() -> (w80:bool)
            n981 = Select(t=w79, s=w80, f=w78) -> (s? t:f=w81:u16)
          }
          frame True {
            w82 = u16 0 items=["System  Error", "System Running", "System Standby"] ("System Status")
          }
        }
        n982 = local read "Stop"() -> (w77:bool)
        n983 = local write "System Status"(w74) -> ()
      }
      n984 = while {
        tunnel: w61 -> [w83]
        stop <- w89 stop-if-true
        n985 = call-poly <vilib>:"Analog Read.vi"("Analog Channel"=u8 0, "LINX Resource"=w83) -> ("Voltage"=w84:dbl)  [unwired: 6 in, 3 out]
        "Phase_Sensor_voltage" <- w84
        n986 = Wait (ms)(milliseconds to wait=u32 300) -> ()  [unwired: 1 out]
        n987 = Build Array(w84) -> (w86:dbl[])
        n988 = Array To Cluster(array=w86) -> (cluster=→"Phase Sensor Chart":T3)
        n989 = local read "Stop"() -> (w89:bool)
      }
      n990 = while {
        stop <- w71 stop-if-true
        n991 = script code="TempArrLED=circshift(TempArrLED,9);\nTempArrLED(10)=T1;\navgTemp = mean(TempArrLED);"() -> ("avgTemp"=w67:dbl)  [unwired: 1 in, 1 out]
        n992 = Wait (ms)(milliseconds to wait=u32 1000) -> ()  [unwired: 1 out]
        n993 = Greater?(x=w67, y=110.0) -> (0:w69:bool)
        n994 = case shown="True" w69 {
          frame False {
          }
          frame True {
            w73 = TRUE
            n995 = local write "Stop"(w73) -> ()
            n996 = local write "System Error"(w73) -> ()
            n997 = local write "Error Message"("Temperature in Bay 2 is above 110'C") -> ()
            n998 = script code="system_error = 1;"() -> ()  [unwired: 1 in, 1 out]
          }
        }
        n999 = local read "Stop"() -> (w71:bool)
      }
      n1000 = while {
        tunnel: w61 -> [w102]
        stop <- w127 stop-if-true
        w109 = 270
        w103 = 600
        w104 = 600
        # "Read Pressure and Flowrate"
        n1001 = local read "Stop"() -> (w127:bool)
        n1002 = call-poly <vilib>:"Analog Read.vi"("AI Channel(s)"=i32[] [14, 15, 14, 15], "LINX Resource"=w102) -> ("Voltages"=w100:dbl[])  [unwired: 6 in, 3 out]
        n1003 = Index Array(array=w100, index=1) -> (element=w123:dbl)
        n1004 = Index Array(array=w100, index=0) -> (element=w124:dbl)
        n1005 = call-poly <vilib>:"PID Control Input Filter.vi"("input"=w123) -> ("output"=w116:dbl)  [unwired: 4 in]
        n1006 = call-poly <vilib>:"PID Control Input Filter.vi"("input"=w124) -> ("output"=w115:dbl)  [unwired: 4 in]
        n1007 = Multiply(x=104.96 ("y"), y=w116) -> (x*y=w117:dbl)
        n1008 = Multiply(x=104.96 ("y"), y=w115) -> (x*y=w120:dbl)
        n1009 = Subtract(x=w117, y=24.077) -> (x-y=w107:dbl)
        n1010 = Subtract(x=w120, y=24.077) -> (x-y=w108:dbl)
        n1011 = Build Array(w104, w103) -> (w112:i32[])
        n1012 = Array To Cluster(array=w112) -> (cluster=→"Flowrate Chart":T4)
        n1013 = Build Array(w108, w107) -> (w113:dbl[])
        n1014 = local write "Flowrate Sensor 1"(w104) -> ()
        n1015 = local write "Flowrate Sensor 2"(w103) -> ()
        n1016 = local write "Pressure 1"(w108) -> ()
        n1017 = local write "Pressure 2"(w107) -> ()
        n1018 = Array To Cluster(array=w113) -> (cluster=→"Pressure Chart":T3)
        n1019 = Wait (ms)(milliseconds to wait=u32 500) -> ()  [unwired: 1 out]
        n1020 = script code="MATLAB script"("F1"=w104, "F2"=w103, "Pres1"=w108, "Pres2"=w107) -> ()  [unwired: 1 in, 1 out]
        n1021 = Greater?(x=w107, y=w109) -> (0:w105:bool)
        n1022 = Greater?(x=w108, y=w109) -> (0:w106:bool)
        n1023 = case shown="False" w106 {
          frame False {
          }
          frame True {
            w131 = TRUE ("Stop")
            n1024 = local write "System Error"(w131) -> ()
            n1025 = local write "Stop"(w131) -> ()
            n1026 = local write "Error Message"("Pressure Sensor 1 readings above 250psi") -> ()
            n1027 = script code="system_error = 1;"() -> ()  [unwired: 1 in, 1 out]
          }
        }
        n1028 = case shown="True" w105 {
          frame False {
          }
          frame True {
            w129 = TRUE ("Stop")
            n1029 = local write "System Error"(w129) -> ()
            n1030 = local write "Error Message"("Pressure Sensor 2 readings above 250psi") -> ()
            n1031 = local write "Stop"(w129) -> ()
            n1032 = script code="system_error = 1;"() -> ()  [unwired: 1 in, 1 out]
          }
        }
      }
    }
    frame #3 {
      # "Save and close xml and excel file"
      n1033 = script code="if exist('xl_file','var') & exist('xlApp','var')\n  xlWorkbook.SaveAs(xl_file);\n  xlWorkbook.Close;\n  xlApp.Quit;\n  xlApp.delete;\nend"() -> ()  [unwired: 1 in, 1 out]
    }
    frame #4 {
      w1385 = string[] ["e", "f", "g", "h", "i", "j"]
      # "End communication to hardware"
      n1034 = local read "Syringe_pump?"() -> (w1383:bool)
      n1035 = local read "COMM Port:: Harvard Syringe Pump"() -> (w1384:refnum<visa-resource-name>)
      n1036 = local read "IR Sensor Device"() -> (w1382:T6)
      n1037 = local read "COMM Port :: Milligat Pumps"() -> (w1387:refnum<visa-resource-name>)
      n1038 = call <vilib>:"Close.vi"("LINX Resource"=w1381) -> ()  [unwired: 10 in, 1 out]
      n1039 = Array Size(array=w1385) -> (size(s)=w1386:i32)
      n1040 = case shown="True" w1383 {
        tunnel: w1384 -> [_ w1388]
        frame False {
        }
        frame True {
          n1041 = call <instrlib>:"Stop Pump.vi"("VISA resource name"=w1388) -> ()  [unwired: 9 in, 2 out]
        }
      }
      n1042 = for {
        N: w1386 -> [_]
        tunnel: w1385 -> [w1389] mode=indexing
        tunnel: w1387 -> [w1390]
        n1043 = call "PumpStop.vi"("Pump Address"=w1389, "Pump COMM Port"=w1390) -> ()  [unwired: 9 in, 1 out]
        n1044 = Wait (ms)(milliseconds to wait=u32 300) -> ()  [unwired: 1 out]
      }
      n1045 = call-poly <vilib>:"NI-845x Close Reference.vi"("device reference"=w1382) -> ()  [unwired: 10 in, 1 out]
    }
    frame #5 {
      # "Display Error Messages if necessary"
      n1046 = local read "Error Message"() -> (w1392:string)
      n1047 = One Button Dialog(message=w1392) -> ()  [unwired: 1 in, 1 out]
    }
  }
